vi "error_ checker.vi"() -> ()   [LabVIEW 2017]
uses:
  <vilib>/FPGAPlugInAG/myRIO-1900/niLvFpga_Open_myRIO-1900.vi
  <vilib>/rvi/interface/common/dynamic/niFpgaDynamicAddResources.vi
  <vilib>/rvi/interface/common/niFpgaWaitOnOcc.vi
  <vilib>/Utility/error.llb/Error Cluster From Error Code.vi
  <vilib>/rvi/errors/niLvFpgaAdjustHostInterfaceError.vi
  <vilib>/express/express shared/transition.llb/Dynamic To Waveform Array.vi
  <vilib>/express/express signal manip/GetorSetDDTAttributes/Set DDT Attributes/SetT0.vi
  <vilib>/express/express shared/transition.llb/Waveform Array To Dynamic.vi
  <vilib>/FPGAPlugInAG/Dynamic/niLvFpga_Close_Dynamic.vi
  <vilib>/rvi/interface/nirviOpenFPGA/nirviOpenFPGA.xnode
  FPGA Bitfiles/testznakowarki_FPGATarget_readtescior_VLrWmtzxVOU.lvbitx
  read_and_write.vi
  <vilib>/rvi/interface/nirviMethod/nirviMethod.xnode
  <vilib>/rvi/interface/nirviReadWriteControl/nirviReadWriteControl.xnode
  <vilib>/express/express signal manip/GetorSetDDTAttributes/Set DDT Attributes/Set DDT Properties.xnode
  <vilib>/rvi/interface/nirviCloseFPGA/nirviCloseFPGA.xnode
  <vilib>/rvi/errors/niLvFpgaMergeErrorWithErrorCode.vi
  <vilib>/FPGAPlugInAG/Dynamic/niLvFpga_ConfigureFifo_Dynamic.vi
  NiFpgaLv.dll
  <vilib>/rvi/interface/Simulation/niFpgaSimulationCallBeginRW.vi
  <vilib>/FPGAPlugInAG/Dynamic/niLvFpga_ReadFifo_Dynamic.vi
panel:
  in  "stop":bool
  out "?":string="this parameter determines how fast function reads data, higher value means slower reading and lower accuracy (use hundreds or thousands)"
  in  "ticks reading":u32=500
  out "Warning":string="cannot exceed 1023 and must be lower than number of pts after trigger stops (better not go under 150)"
  in  "number of elements":u32=150
  out "cycles to complete":i32
  out "gen size checker":i32
  in  "?":enum32{"now", "data", "settings"}(tab)=enum."settings"
  out "gathered error x graph":cluster{"time":i32[], "data y":i16[]}[](graph)=[{"time"=[0, 1, 2, 3, 4, 5, 6, 7, 8, 9, 10, 11, 12, 13, 14, 15, 16, 17, 18, 19, 20, 21, 22, 23, 24, 25, 26, 27, 28, 29, 30, 31, 32, 33, 34, 35, 36, 37, 38, 39, 40, 41, 42, 43, 44, 45, 46, 47, 48, 49, 50, 51, 52, 53, 54, 55, 56, 57, 58, 59, 60, 61, 62, 63, 64, 65, 66, 67, 68, 69, 70, 71, 72, 73, 74, 75, 76, 77, 78, 79, 80, 81, 82, 83, 84, 85, 86, 87, 88, 89, 90, 91, 92, 93, 94, 95, 96, 97, 98, 99, 100, 101, 102, 103, 104, 105, 106, 107, 108, 109, 110, 111, 112, 113, 114, 115, 116, 117, 118, 119, 120, 121, 122, 123, 124, 125, 126, 127, 128, 129, 130, 131, 132, 133, 134, 135, 136, 137, 138, 139, 140, 141, 142, 143, 144, 145, 146, 147, 148, 149, 150, 151, 152, 153, 154, 155, 156, 157, 158, 159, 160, 161, 162, 163, 164, 165, 166, 167, 168, 169, 170, 171, 172, 173, 174, 175, 176, 177, 178, 179, 180, 181, 182, 183, 184, 185, 186, 187, 188, 189, 190, 191, 192, 193, 194, 195, 196, 197, 198, 199, 200, 201, 202, 203, 204, 205, 206, 207, 208, 209, 210, 211, 212, 213, 214, 215, 216, 217, 218, 219, 220, 221, 222, 223, 224, 225, 226, 227, 228, 229, 230, 231, 232, 233, 234, 235, 236, 237, 238, 239, 240, 241, 242, 243, 244, 245, 246, 247, 248, 249, 250, 251, 252, 253, 254, 255, 256, 257, 258, 259, 260, 261, 262, 263, 264, 265, 266, 267, 268, 269, 270, 271, 272, 273, 274, 275, 276, 277, 278, 279, 280, 281, 282, 283, 284, 285, 286, 287, 288, 289, 290, 291, 292, 293, 294, 295, 296, 297, 298, 299], "data y"=[1986, 1970, 1920, 1858, 1861, 1860, 1808, 1774, 1734, 1748, 1695, 1675, 1665, 1650, 1668, 1624, 1652, 1624, 1636, 1627, 1647, 1655, 1677, 1675, 1696, 1728, 1732, 1725, 1767, 1796, 1796, 1846, 1885, 1873, 1909, 1930, 1975, 1952, 1993, 2008, 2014, 1986, 2017, 2037, 2018, 2020, 2017, 1998, 1997, 2030, 2037, 2018, 2013, 2029, 2019, 2007, 2043, 2014, 2019, 2007, 2050, 2067, 1998, 1985, 2043, 2057, 2007, 1991, 1987, 2004, 2037, 2047, 2025, 2039, 2020, 2050, 2026, 2017, 2027, 1996, 1995, 2047, 2055, 2019, 2007, 2022, 2029, 1994, 2029, 2067, 2028, 2005, 2024, 2042, 2033, 2047, 2027, 2005, 2016, 2041, 2018, 2017, 2008, 2015, 2025, 2052, 2056, 2042, 2049, 2011, 2005, 2043, 2052, 2027, 2021, 2058, 2051, 2038, 2045, 2022, 2015, 2048, 2058, 2047, 2061, 2024, 2039, 2035, 2055, 2055, 2022, 2037, 2039, 2014, 2036, 2053, 2025, 2054, 2042, 2058, 2034, 2044, 2063, 2042, 2023, 2043, 2027, 2039, 2067, 2063, 2047, 2011, 2045, 2057, 2037, 2051, 2049, 2016, 2038, 2064, 2038, 2041, 2053, 2027, 2045, 2040, 2064, 2037, 2020, 2047, 2047, 2032, 2068, 2049, 2023, 2035, 2043, 2081, 2038, 2041, 2045, 2010, 2028, 2059, 2045, 2050, 2067, 2035, 2035, 2059, 2051, 2040, 2025, 2051, 2052, 2031, 2063, 2062, 2027, 2051, 2054, 2022, 2036, 2040, 2057, 2037, 2048, 2064, 2038, 2033, 2058, 2045, 2037, 2051, 2027, 2053, 2025, 2031, 2033, 2023, 2049, 2053, 2038, 2054, 2050, 2025, 2041, 2067, 2039, 2016, 2030, 2056, 2045, 2052, 2067, 2029, 2027, 2045, 2023, 2031, 2065, 2065, 2053, 2041, 2057, 2037, 2017, 2027, 2027, 2028, 2064, 2078, 2042, 2045, 2036, 2069, 2043, 2032, 2038, 2018, 2047, 2072, 2041, 2045, 2053, 2026, 2030, 2016, 2034, 2023, 2025, 2065, 2047, 2029, 2041, 2029, 2032, 2067, 2054, 2031, 2051, 2067, 2051, 2016, 2036, 2063, 2047, 2060, 2064, 2026, 2024, 2045, 2026, 2028, 2012, 2034, 2026, 2031, 2055, 2041]}, {"time"=[0, 1, 2, 3, 4, 5, 6, 7, 8, 9, 10, 11, 12, 13, 14, 15, 16, 17, 18, 19, 20, 21, 22, 23, 24, 25, 26, 27, 28, 29, 30, 31, 32, 33, 34, 35, 36, 37, 38, 39, 40, 41, 42, 43, 44, 45, 46, 47, 48, 49, 50, 51, 52, 53, 54, 55, 56, 57, 58, 59, 60, 61, 62, 63, 64, 65, 66, 67, 68, 69, 70, 71, 72, 73, 74, 75, 76, 77, 78, 79, 80, 81, 82, 83, 84, 85, 86, 87, 88, 89, 90, 91, 92, 93, 94, 95, 96, 97, 98, 99, 100, 101, 102, 103, 104, 105, 106, 107, 108, 109, 110, 111, 112, 113, 114, 115, 116, 117, 118, 119, 120, 121, 122, 123, 124, 125, 126, 127, 128, 129, 130, 131, 132, 133, 134, 135, 136, 137, 138, 139, 140, 141, 142, 143, 144, 145, 146, 147, 148, 149, 150, 151, 152, 153, 154, 155, 156, 157, 158, 159, 160, 161, 162, 163, 164, 165, 166, 167, 168, 169, 170, 171, 172, 173, 174, 175, 176, 177, 178, 179, 180, 181, 182, 183, 184, 185, 186, 187, 188, 189, 190, 191, 192, 193, 194, 195, 196, 197, 198, 199, 200, 201, 202, 203, 204, 205, 206, 207, 208, 209, 210, 211, 212, 213, 214, 215, 216, 217, 218, 219, 220, 221, 222, 223, 224, 225, 226, 227, 228, 229, 230, 231, 232, 233, 234, 235, 236, 237, 238, 239, 240, 241, 242, 243, 244, 245, 246, 247, 248, 249, 250, 251, 252, 253, 254, 255, 256, 257, 258, 259, 260, 261, 262, 263, 264, 265, 266, 267, 268, 269, 270, 271, 272, 273, 274, 275, 276, 277, 278, 279, 280, 281, 282, 283, 284, 285, 286, 287, 288, 289, 290, 291, 292, 293, 294, 295, 296, 297, 298, 299], "data y"=[2382, 2659, 2664, 2672, 2666, 2654, 2660, 2664, 2667, 2655, 2663, 2668, 2662, 2667, 2660, 2658, 2661, 2670, 2657, 2659, 2671, 2214, 1624, 1315, 1097, 961, 861, 782, 703, 622, 628, 628, 621, 632, 635, 636, 668, 754, 892, 1012, 1172, 1362, 1513, 1661, 1801, 1899, 1955, 2029, 2076, 2101, 2109, 2111, 2110, 2082, 2059, 2050, 2019, 2037, 2053, 2067, 2089, 2092, 2091, 2116, 2097, 2066, 2077, 2087, 2092, 2091, 2075, 2066, 2058, 2046, 2042, 2030, 2048, 2065, 2051, 2053, 2073, 2052, 2041, 2052, 2058, 2057, 2062, 2070, 2067, 2039, 2044, 2048, 2041, 2035, 2026, 2037, 2059, 2060, 2064, 2055, 2051, 2045, 2046, 2067, 2066, 2040, 2041, 2052, 2045, 2056, 2059, 2044, 2042, 2049, 2042, 2045, 2048, 2064, 2060, 2052, 2064, 2055, 2049, 2055, 2038, 2049, 2038, 2059, 2059, 2059, 2053, 2052, 2046, 2056, 2051, 2029, 2043, 2048, 2054, 2041, 2058, 2056, 2039, 2045, 2065, 2054, 2055, 2056, 2040, 2049, 2055, 2052, 2042, 2044, 2058, 2064, 2055, 2068, 2065, 2050, 2052, 2058, 2039, 2040, 2037, 2050, 2054, 2060, 2067, 2043, 2053, 2057, 2047, 2037, 2050, 2054, 2047, 2035, 2047, 2063, 2052, 2061, 2064, 2047, 2055, 2066, 2056, 2062, 2068, 2061, 2042, 2035, 2047, 2037, 2034, 2043, 2046, 2039, 2053, 2058, 2051, 2070, 2063, 2056, 2042, 2055, 2069, 2039, 2044, 2052, 2049, 2048, 2061, 2059, 2057, 2043, 2058, 2052, 2041, 2054, 2044, 2038, 2048, 2045, 2043, 2072, 2072, 2057, 2058, 2056, 2063, 2049, 2054, 2056, 2047, 2046, 2059, 2041, 2042, 2055, 2052, 2045, 2045, 2059, 2050, 2057, 2068, 2054, 2051, 2057, 2041, 2031, 2051, 2048, 2056, 2040, 2050, 2056, 2045, 2062, 2059, 2035, 2032, 2053, 2042, 2056, 2063, 2063, 2048, 2052, 2065, 2057, 2044, 2053, 2053, 2043, 2050, 2058, 2035, 2058, 2049, 2058, 2047, 2056, 2061, 2045, 2052, 2054, 2042, 2051, 2051, 2056, 2062, 2047, 2066, 2048, 2050, 2062, 2056, 2049]}]
  out "gathered error y graph":cluster{"time":i32[], "data y":i16[]}[](graph)=[{"time"=[0, 1, 2, 3, 4, 5, 6, 7, 8, 9, 10, 11, 12, 13, 14, 15, 16, 17, 18, 19, 20, 21, 22, 23, 24, 25, 26, 27, 28, 29, 30, 31, 32, 33, 34, 35, 36, 37, 38, 39, 40, 41, 42, 43, 44, 45, 46, 47, 48, 49, 50, 51, 52, 53, 54, 55, 56, 57, 58, 59, 60, 61, 62, 63, 64, 65, 66, 67, 68, 69, 70, 71, 72, 73, 74, 75, 76, 77, 78, 79, 80, 81, 82, 83, 84, 85, 86, 87, 88, 89, 90, 91, 92, 93, 94, 95, 96, 97, 98, 99, 100, 101, 102, 103, 104, 105, 106, 107, 108, 109, 110, 111, 112, 113, 114, 115, 116, 117, 118, 119, 120, 121, 122, 123, 124, 125, 126, 127, 128, 129, 130, 131, 132, 133, 134, 135, 136, 137, 138, 139, 140, 141, 142, 143, 144, 145, 146, 147, 148, 149, 150, 151, 152, 153, 154, 155, 156, 157, 158, 159, 160, 161, 162, 163, 164, 165, 166, 167, 168, 169, 170, 171, 172, 173, 174, 175, 176, 177, 178, 179, 180, 181, 182, 183, 184, 185, 186, 187, 188, 189, 190, 191, 192, 193, 194, 195, 196, 197, 198, 199, 200, 201, 202, 203, 204, 205, 206, 207, 208, 209, 210, 211, 212, 213, 214, 215, 216, 217, 218, 219, 220, 221, 222, 223, 224, 225, 226, 227, 228, 229, 230, 231, 232, 233, 234, 235, 236, 237, 238, 239, 240, 241, 242, 243, 244, 245, 246, 247, 248, 249, 250, 251, 252, 253, 254, 255, 256, 257, 258, 259, 260, 261, 262, 263, 264, 265, 266, 267, 268, 269, 270, 271, 272, 273, 274, 275, 276, 277, 278, 279, 280, 281, 282, 283, 284, 285, 286, 287, 288, 289, 290, 291, 292, 293, 294, 295, 296, 297, 298, 299], "data y"=[2052, 2061, 2063, 2041, 2035, 2058, 2066, 2066, 2068, 2062, 2054, 2045, 2073, 2074, 2031, 2080, 2051, 2055, 2053, 2054, 2043, 2050, 2071, 2049, 2039, 2046, 2056, 2052, 2059, 2073, 2060, 2061, 2059, 2053, 2058, 2041, 2063, 2064, 2041, 2074, 2068, 2060, 2061, 2064, 2053, 2064, 2069, 2050, 2057, 2054, 2058, 2068, 2050, 2066, 2058, 2050, 2048, 2081, 2035, 2068, 2067, 2055, 2041, 2070, 2087, 2039, 2024, 2054, 2084, 2074, 2072, 2075, 2054, 2050, 2042, 2059, 2070, 2058, 2070, 2066, 2030, 2041, 2074, 2068, 2051, 2046, 2038, 2042, 2033, 2063, 2075, 2051, 2043, 2045, 2055, 2072, 2070, 2055, 2048, 2075, 2054, 2057, 2058, 2055, 2044, 2046, 2064, 2059, 2068, 2056, 2038, 2052, 2062, 2062, 2038, 2053, 2076, 2054, 2060, 2063, 2037, 2046, 2061, 2046, 2058, 2035, 2053, 2046, 2052, 2063, 2052, 2047, 2059, 2040, 2038, 2060, 2050, 2050, 2053, 2059, 2052, 2039, 2063, 2065, 2052, 2055, 2054, 2039, 2056, 2066, 2056, 2029, 2034, 2060, 2058, 2056, 2072, 2053, 2039, 2055, 2052, 2045, 2060, 2057, 2065, 2049, 2063, 2074, 2046, 2047, 2055, 2032, 2047, 2072, 2051, 2051, 2066, 2072, 2070, 2051, 2059, 2046, 2032, 2047, 2057, 2052, 2073, 2073, 2049, 2057, 2053, 2063, 2048, 2046, 2064, 2046, 2057, 2075, 2056, 2049, 2067, 2045, 2041, 2046, 2059, 2061, 2046, 2060, 2055, 2037, 2051, 2062, 2055, 2063, 2060, 2080, 2051, 2046, 2047, 2029, 2038, 2060, 2054, 2060, 2074, 2052, 2047, 2053, 2057, 2048, 2032, 2054, 2054, 2047, 2064, 2059, 2037, 2043, 2051, 2044, 2065, 2045, 2059, 2050, 2065, 2071, 2047, 2042, 2047, 2033, 2042, 2064, 2058, 2053, 2031, 2065, 2064, 2049, 2059, 2047, 2044, 2053, 2059, 2053, 2069, 2059, 2033, 2041, 2045, 2053, 2035, 2046, 2064, 2045, 2051, 2058, 2041, 2052, 2068, 2054, 2055, 2060, 2071, 2055, 2038, 2060, 2052, 2047, 2069, 2058, 2042, 2056, 2049, 2066, 2040, 2050, 2056, 2034, 2055, 2059]}, {"time"=[0, 1, 2, 3, 4, 5, 6, 7, 8, 9, 10, 11, 12, 13, 14, 15, 16, 17, 18, 19, 20, 21, 22, 23, 24, 25, 26, 27, 28, 29, 30, 31, 32, 33, 34, 35, 36, 37, 38, 39, 40, 41, 42, 43, 44, 45, 46, 47, 48, 49, 50, 51, 52, 53, 54, 55, 56, 57, 58, 59, 60, 61, 62, 63, 64, 65, 66, 67, 68, 69, 70, 71, 72, 73, 74, 75, 76, 77, 78, 79, 80, 81, 82, 83, 84, 85, 86, 87, 88, 89, 90, 91, 92, 93, 94, 95, 96, 97, 98, 99, 100, 101, 102, 103, 104, 105, 106, 107, 108, 109, 110, 111, 112, 113, 114, 115, 116, 117, 118, 119, 120, 121, 122, 123, 124, 125, 126, 127, 128, 129, 130, 131, 132, 133, 134, 135, 136, 137, 138, 139, 140, 141, 142, 143, 144, 145, 146, 147, 148, 149, 150, 151, 152, 153, 154, 155, 156, 157, 158, 159, 160, 161, 162, 163, 164, 165, 166, 167, 168, 169, 170, 171, 172, 173, 174, 175, 176, 177, 178, 179, 180, 181, 182, 183, 184, 185, 186, 187, 188, 189, 190, 191, 192, 193, 194, 195, 196, 197, 198, 199, 200, 201, 202, 203, 204, 205, 206, 207, 208, 209, 210, 211, 212, 213, 214, 215, 216, 217, 218, 219, 220, 221, 222, 223, 224, 225, 226, 227, 228, 229, 230, 231, 232, 233, 234, 235, 236, 237, 238, 239, 240, 241, 242, 243, 244, 245, 246, 247, 248, 249, 250, 251, 252, 253, 254, 255, 256, 257, 258, 259, 260, 261, 262, 263, 264, 265, 266, 267, 268, 269, 270, 271, 272, 273, 274, 275, 276, 277, 278, 279, 280, 281, 282, 283, 284, 285, 286, 287, 288, 289, 290, 291, 292, 293, 294, 295, 296, 297, 298, 299], "data y"=[2038, 2035, 2029, 2040, 2046, 2033, 2032, 2044, 2045, 2051, 2047, 2071, 2062, 2041, 2051, 2057, 2045, 2056, 2044, 2031, 2045, 2055, 2077, 2043, 2027, 2024, 2008, 2031, 2040, 2035, 2041, 2047, 2038, 2036, 2058, 2071, 2043, 2042, 2051, 2057, 2038, 2058, 2064, 2032, 2042, 2053, 2038, 2035, 2028, 2043, 2031, 2041, 2046, 2044, 2028, 2042, 2034, 2027, 2025, 2040, 2014, 2026, 2051, 2058, 2041, 2044, 2072, 2066, 2044, 2037, 2040, 2038, 2050, 2052, 2053, 2048, 2038, 2045, 2049, 2031, 2056, 2055, 2035, 2034, 2051, 2053, 2052, 2037, 2060, 2043, 2027, 2029, 2040, 2037, 2028, 2041, 2035, 2024, 2049, 2039, 2034, 2036, 2030, 2050, 2050, 2042, 2036, 2041, 2036, 2038, 2041, 2030, 2043, 2044, 2053, 2056, 2047, 2055, 2049, 2029, 2034, 2048, 2041, 2044, 2050, 2044, 2036, 2047, 2050, 2022, 2023, 2032, 2040, 2034, 2051, 2043, 2039, 2044, 2052, 2049, 2040, 2048, 2033, 2021, 2034, 2032, 2026, 2049, 2051, 2034, 2049, 2054, 2055, 2045, 2049, 2058, 2048, 2048, 2057, 2047, 2044, 2046, 2037, 2032, 2044, 2043, 2042, 2032, 2034, 2048, 2045, 2053, 2054, 2031, 2015, 2032, 2032, 2030, 2030, 2033, 2039, 2045, 2062, 2048, 2044, 2052, 2047, 2027, 2037, 2043, 2049, 2047, 2051, 2046, 2033, 2036, 2036, 2037, 2042, 2055, 2035, 2032, 2038, 2037, 2035, 2038, 2060, 2053, 2043, 2046, 2047, 2045, 2048, 2042, 2041, 2026, 2028, 2049, 2045, 2045, 2052, 2041, 2038, 2036, 2027, 2029, 2047, 2045, 2034, 2051, 2081, 2094, 2083, 2101, 2093, 2078, 2070, 2061, 2036, 2027, 2027, 2036, 2012, 2002, 2022, 2018, 2024, 2027, 2021, 2021, 2036, 2025, 2035, 2036, 2026, 2039, 2024, 2029, 2031, 2039, 2062, 2048, 2038, 2039, 2042, 2041, 2055, 2036, 2039, 2029, 2045, 2055, 2034, 2033, 2041, 2037, 2056, 2052, 2037, 2027, 2027, 2038, 2036, 2038, 2050, 2061, 2054, 2046, 2028, 2029, 2036, 2040, 2034, 2027, 2028, 2037, 2025, 2050, 2048, 2041]}]
  out "error x graph current elements":cluster{"time":i32[], "data y":i16[]}[](graph)=[{"time"=[0, 1, 2, 3, 4, 5, 6, 7, 8, 9, 10, 11, 12, 13, 14, 15, 16, 17, 18, 19, 20, 21, 22, 23, 24, 25, 26, 27, 28, 29, 30, 31, 32, 33, 34, 35, 36, 37, 38, 39, 40, 41, 42, 43, 44, 45, 46, 47, 48, 49, 50, 51, 52, 53, 54, 55, 56, 57, 58, 59, 60, 61, 62, 63, 64, 65, 66, 67, 68, 69, 70, 71, 72, 73, 74, 75, 76, 77, 78, 79, 80, 81, 82, 83, 84, 85, 86, 87, 88, 89, 90, 91, 92, 93, 94, 95, 96, 97, 98, 99, 100, 101, 102, 103, 104, 105, 106, 107, 108, 109, 110, 111, 112, 113, 114, 115, 116, 117, 118, 119, 120, 121, 122, 123, 124, 125, 126, 127, 128, 129, 130, 131, 132, 133, 134, 135, 136, 137, 138, 139, 140, 141, 142, 143, 144, 145, 146, 147, 148, 149], "data y"=[2071, 2039, 2036, 2051, 2051, 2040, 2029, 2062, 2055, 2035, 2053, 2044, 2025, 2060, 2073, 2030, 2042, 2039, 2050, 2027, 2018, 2046, 2065, 2037, 2057, 2053, 2030, 2049, 2072, 2034, 2032, 2069, 2083, 2035, 2030, 2040, 2024, 2055, 2070, 2033, 2041, 2049, 2031, 2029, 2032, 2062, 2045, 2038, 2054, 2026, 2016, 2048, 2049, 2056, 2084, 2060, 2040, 2028, 2066, 2074, 2043, 2052, 2055, 2015, 2037, 2057, 2029, 2048, 2069, 2071, 2045, 2044, 2061, 2031, 2028, 2050, 2031, 2019, 2047, 2042, 2042, 2005, 2029, 2053, 2044, 2072, 2074, 2039, 2044, 2049, 2016, 2032, 2063, 2045, 2044, 2043, 2073, 2063, 2043, 2058, 2045, 2025, 2047, 2057, 2042, 2063, 2066, 2051, 2019, 2033, 2062, 2055, 2062, 2069, 2033, 2017, 2035, 2015, 2027, 2069, 2055, 2051, 2026, 2055, 2066, 2026, 2042, 2049, 2025, 2052, 2074, 2037, 2052, 2032, 2052, 2038, 2035, 2071, 2063, 2047, 2063, 2041, 2011, 2026, 2048, 2036, 2023, 2027, 2061, 2046]}, {"time"=[0, 1, 2, 3, 4, 5, 6, 7, 8, 9, 10, 11, 12, 13, 14, 15, 16, 17, 18, 19, 20, 21, 22, 23, 24, 25, 26, 27, 28, 29, 30, 31, 32, 33, 34, 35, 36, 37, 38, 39, 40, 41, 42, 43, 44, 45, 46, 47, 48, 49, 50, 51, 52, 53, 54, 55, 56, 57, 58, 59, 60, 61, 62, 63, 64, 65, 66, 67, 68, 69, 70, 71, 72, 73, 74, 75, 76, 77, 78, 79, 80, 81, 82, 83, 84, 85, 86, 87, 88, 89, 90, 91, 92, 93, 94, 95, 96, 97, 98, 99, 100, 101, 102, 103, 104, 105, 106, 107, 108, 109, 110, 111, 112, 113, 114, 115, 116, 117, 118, 119, 120, 121, 122, 123, 124, 125, 126, 127, 128, 129, 130, 131, 132, 133, 134, 135, 136, 137, 138, 139, 140, 141, 142, 143, 144, 145, 146, 147, 148, 149], "data y"=[2031, 2054, 2044, 2020, 2028, 2026, 2038, 2032, 2038, 2052, 2051, 2045, 2052, 2046, 2035, 2047, 2043, 2036, 2028, 2038, 2051, 2042, 2033, 2029, 2035, 2043, 2060, 2055, 2033, 2037, 2044, 2041, 2039, 2042, 2048, 2039, 2050, 2042, 2030, 2039, 2042, 2034, 2037, 2048, 2059, 2039, 2035, 2035, 2032, 2041, 2051, 2038, 2036, 2039, 2045, 2042, 2042, 2049, 2028, 2031, 2036, 2041, 2048, 2056, 2048, 2025, 2034, 2037, 2026, 2042, 2045, 2058, 2040, 2028, 2043, 2033, 2039, 2064, 2056, 2046, 2052, 2042, 2039, 2027, 2041, 2048, 2036, 2049, 2056, 2047, 2047, 2043, 2028, 2039, 2046, 2058, 2039, 2033, 2035, 2035, 2033, 2043, 2035, 2040, 2053, 2050, 2049, 2045, 2044, 2051, 2030, 2038, 2051, 2038, 2047, 2050, 2040, 2047, 2055, 2033, 2055, 2049, 2049, 2041, 2033, 2045, 2042, 2033, 2050, 2058, 2042, 2049, 2050, 2049, 2036, 2041, 2047, 2039, 2041, 2053, 2036, 2043, 2053, 2048, 2040, 2050, 2049, 2055, 2042, 2037]}]
  out "error y graph current elements":cluster{"time":i32[], "data y":i16[]}[](graph)=[{"time"=[0, 1, 2, 3, 4, 5, 6, 7, 8, 9, 10, 11, 12, 13, 14, 15, 16, 17, 18, 19, 20, 21, 22, 23, 24, 25, 26, 27, 28, 29, 30, 31, 32, 33, 34, 35, 36, 37, 38, 39, 40, 41, 42, 43, 44, 45, 46, 47, 48, 49, 50, 51, 52, 53, 54, 55, 56, 57, 58, 59, 60, 61, 62, 63, 64, 65, 66, 67, 68, 69, 70, 71, 72, 73, 74, 75, 76, 77, 78, 79, 80, 81, 82, 83, 84, 85, 86, 87, 88, 89, 90, 91, 92, 93, 94, 95, 96, 97, 98, 99, 100, 101, 102, 103, 104, 105, 106, 107, 108, 109, 110, 111, 112, 113, 114, 115, 116, 117, 118, 119, 120, 121, 122, 123, 124, 125, 126, 127, 128, 129, 130, 131, 132, 133, 134, 135, 136, 137, 138, 139, 140, 141, 142, 143, 144, 145, 146, 147, 148, 149], "data y"=[2068, 2051, 2035, 2052, 2049, 2060, 2029, 2046, 2069, 2056, 2055, 2055, 2034, 2045, 2070, 2055, 2046, 2047, 2067, 2061, 2039, 2034, 2051, 2048, 2059, 2067, 2047, 2037, 2058, 2053, 2044, 2042, 2066, 2060, 2043, 2052, 2037, 2041, 2051, 2043, 2030, 2050, 2044, 2054, 2036, 2047, 2055, 2042, 2056, 2057, 2036, 2045, 2054, 2043, 2057, 2072, 2051, 2030, 2044, 2068, 2059, 2056, 2065, 2042, 2029, 2050, 2042, 2040, 2065, 2054, 2061, 2038, 2053, 2055, 2032, 2055, 2061, 2039, 2046, 2053, 2030, 2036, 2029, 2049, 2043, 2052, 2074, 2061, 2048, 2058, 2043, 2028, 2047, 2053, 2057, 2039, 2049, 2063, 2043, 2056, 2063, 2047, 2046, 2059, 2049, 2050, 2059, 2060, 2049, 2034, 2049, 2053, 2047, 2070, 2063, 2039, 2041, 2042, 2025, 2049, 2052, 2060, 2032, 2037, 2059, 2052, 2039, 2062, 2048, 2041, 2066, 2056, 2037, 2038, 2052, 2060, 2035, 2053, 2072, 2053, 2060, 2068, 2041, 2035, 2049, 2037, 2055, 2034, 2042, 2055]}, {"time"=[0, 1, 2, 3, 4, 5, 6, 7, 8, 9, 10, 11, 12, 13, 14, 15, 16, 17, 18, 19, 20, 21, 22, 23, 24, 25, 26, 27, 28, 29, 30, 31, 32, 33, 34, 35, 36, 37, 38, 39, 40, 41, 42, 43, 44, 45, 46, 47, 48, 49, 50, 51, 52, 53, 54, 55, 56, 57, 58, 59, 60, 61, 62, 63, 64, 65, 66, 67, 68, 69, 70, 71, 72, 73, 74, 75, 76, 77, 78, 79, 80, 81, 82, 83, 84, 85, 86, 87, 88, 89, 90, 91, 92, 93, 94, 95, 96, 97, 98, 99, 100, 101, 102, 103, 104, 105, 106, 107, 108, 109, 110, 111, 112, 113, 114, 115, 116, 117, 118, 119, 120, 121, 122, 123, 124, 125, 126, 127, 128, 129, 130, 131, 132, 133, 134, 135, 136, 137, 138, 139, 140, 141, 142, 143, 144, 145, 146, 147, 148, 149], "data y"=[2036, 2036, 2036, 2027, 2041, 2049, 2053, 2045, 2033, 2036, 2043, 2038, 2041, 2048, 2028, 2040, 2061, 2051, 2042, 2027, 2042, 2055, 2032, 2026, 2042, 2037, 2044, 2064, 2046, 2027, 2053, 2049, 2046, 2037, 2047, 2043, 2044, 2047, 2049, 2045, 2040, 2031, 2039, 2038, 2048, 2055, 2031, 2025, 2025, 2033, 2046, 2051, 2054, 2062, 2044, 2036, 2035, 2046, 2045, 2033, 2038, 2042, 2047, 2053, 2058, 2046, 2052, 2052, 2037, 2051, 2037, 2042, 2043, 2029, 2034, 2039, 2029, 2043, 2049, 2048, 2050, 2035, 2049, 2049, 2043, 2046, 2036, 2040, 2042, 2032, 2033, 2056, 2049, 2019, 2046, 2056, 2058, 2047, 2045, 2045, 2034, 2038, 2048, 2050, 2056, 2054, 2032, 2033, 2038, 2040, 2045, 2035, 2051, 2045, 2031, 2038, 2045, 2042, 2048, 2050, 2057, 2042, 2040, 2054, 2042, 2031, 2038, 2040, 2030, 2051, 2047, 2044, 2060, 2046, 2035, 2026, 2044, 2039, 2042, 2048, 2059, 2053, 2042, 2047, 2051, 2047, 2029, 2049, 2046, 2037]}]
  out "template graph x":cluster{"time":i32[], "data y":i16[]}[](graph)=[{"time"=[0, 1, 2, 3, 4, 5, 6, 7, 8, 9, 10, 11, 12, 13, 14, 15, 16, 17, 18, 19, 20, 21, 22, 23, 24, 25, 26, 27, 28, 29, 30, 31, 32, 33, 34, 35, 36, 37, 38, 39, 40, 41, 42, 43, 44, 45, 46, 47, 48, 49, 50, 51, 52, 53, 54, 55, 56, 57, 58, 59, 60, 61, 62, 63, 64, 65, 66, 67, 68, 69, 70, 71, 72, 73, 74, 75, 76, 77, 78, 79, 80, 81, 82, 83, 84, 85, 86, 87, 88, 89, 90, 91, 92, 93, 94, 95, 96, 97, 98, 99, 100, 101, 102, 103, 104, 105, 106, 107, 108, 109, 110, 111, 112, 113, 114, 115, 116, 117, 118, 119, 120, 121, 122, 123, 124, 125, 126, 127, 128, 129, 130, 131, 132, 133, 134, 135, 136, 137, 138, 139, 140, 141, 142, 143, 144, 145, 146, 147, 148, 149, 150, 151, 152, 153, 154, 155, 156, 157, 158, 159, 160, 161, 162, 163, 164, 165, 166, 167, 168, 169, 170, 171, 172, 173, 174, 175, 176, 177, 178, 179, 180, 181, 182, 183, 184, 185, 186, 187, 188, 189, 190, 191, 192, 193, 194, 195, 196, 197, 198, 199, 200, 201, 202, 203, 204, 205, 206, 207, 208, 209, 210, 211, 212, 213, 214, 215, 216, 217, 218, 219, 220, 221, 222, 223, 224, 225, 226, 227, 228, 229, 230, 231, 232, 233, 234, 235, 236, 237, 238, 239, 240, 241, 242, 243, 244, 245, 246, 247, 248, 249, 250, 251, 252, 253, 254, 255, 256, 257, 258, 259, 260, 261, 262, 263, 264, 265, 266, 267, 268, 269, 270, 271, 272, 273, 274, 275, 276, 277, 278, 279, 280, 281, 282, 283, 284, 285, 286, 287, 288, 289, 290, 291, 292, 293, 294, 295, 296, 297, 298, 299], "data y"=[1987, 1971, 1955, 1885, 1866, 1853, 1810, 1748, 1734, 1732, 1693, 1670, 1650, 1620, 1668, 1631, 1633, 1604, 1653, 1636, 1640, 1666, 1683, 1678, 1678, 1708, 1728, 1718, 1749, 1797, 1795, 1816, 1846, 1904, 1919, 1903, 1949, 1977, 1957, 2028, 2013, 1998, 2012, 2026, 2009, 2022, 2026, 2052, 2031, 2007, 2043, 2018, 2015, 2033, 2040, 1992, 2027, 2023, 2033, 2030, 1985, 2043, 2038, 1979, 2014, 2055, 2048, 2007, 1978, 1979, 2011, 1998, 2018, 2016, 2008, 2028, 2038, 2005, 2018, 2031, 2005, 2038, 2052, 2009, 2023, 2027, 2046, 2020, 2020, 2044, 2019, 2027, 2049, 2016, 2006, 2046, 2025, 2014, 2006, 2032, 2035, 2051, 2066, 2024, 2004, 2035, 2037, 2024, 2053, 2028, 2035, 2032, 2053, 2061, 2024, 2034, 2050, 2011, 2030, 2053, 2036, 2023, 2037, 2053, 2038, 2015, 2038, 2049, 2038, 2057, 2054, 2015, 2040, 2055, 2035, 2017, 2023, 2059, 2050, 2052, 2074, 2039, 2027, 2049, 2031, 2026, 2058, 2069, 2056, 2031, 2058, 2069, 2027, 2018, 2049, 2031, 2034, 2067, 2053, 2042, 2059, 2039, 2051, 2027, 2047, 2065, 2031, 2036, 2064, 2048, 2042, 2060, 2048, 2026, 2027, 2058, 2069, 2034, 2041, 2059, 2032, 2054, 2071, 2037, 2035, 2032, 2034, 2065, 2038, 2032, 2036, 2027, 2025, 2055, 2029, 2029, 2058, 2039, 2033, 2063, 2047, 2035, 2014, 2039, 2033, 2022, 2058, 2042, 2024, 2053, 2049, 2027, 2053, 2041, 2041, 2021, 2048, 2055, 2028, 2045, 2047, 2020, 2031, 2042, 2020, 2027, 2034, 2057, 2036, 2044, 2065, 2026, 2014, 2035, 2030, 2024, 2058, 2040, 2042, 2025, 2048, 2055, 2032, 2042, 2053, 2024, 2042, 2072, 2053, 2054, 2054, 2066, 2045, 2045, 2063, 2039, 2026, 2044, 2030, 2020, 2052, 2039, 2019, 2053, 2034, 2046, 2022, 2057, 2077, 2044, 2045, 2048, 2019, 2031, 2049, 2026, 2027, 2032, 2049, 2029, 2009, 2046, 2052, 2051, 2080, 2061, 2033, 2040, 2029, 2012, 2032, 2044, 2065, 2034, 2037, 2056, 2031, 2042, 2072, 2046]}, {"time"=[0, 1, 2, 3, 4, 5, 6, 7, 8, 9, 10, 11, 12, 13, 14, 15, 16, 17, 18, 19, 20, 21, 22, 23, 24, 25, 26, 27, 28, 29, 30, 31, 32, 33, 34, 35, 36, 37, 38, 39, 40, 41, 42, 43, 44, 45, 46, 47, 48, 49, 50, 51, 52, 53, 54, 55, 56, 57, 58, 59, 60, 61, 62, 63, 64, 65, 66, 67, 68, 69, 70, 71, 72, 73, 74, 75, 76, 77, 78, 79, 80, 81, 82, 83, 84, 85, 86, 87, 88, 89, 90, 91, 92, 93, 94, 95, 96, 97, 98, 99, 100, 101, 102, 103, 104, 105, 106, 107, 108, 109, 110, 111, 112, 113, 114, 115, 116, 117, 118, 119, 120, 121, 122, 123, 124, 125, 126, 127, 128, 129, 130, 131, 132, 133, 134, 135, 136, 137, 138, 139, 140, 141, 142, 143, 144, 145, 146, 147, 148, 149, 150, 151, 152, 153, 154, 155, 156, 157, 158, 159, 160, 161, 162, 163, 164, 165, 166, 167, 168, 169, 170, 171, 172, 173, 174, 175, 176, 177, 178, 179, 180, 181, 182, 183, 184, 185, 186, 187, 188, 189, 190, 191, 192, 193, 194, 195, 196, 197, 198, 199, 200, 201, 202, 203, 204, 205, 206, 207, 208, 209, 210, 211, 212, 213, 214, 215, 216, 217, 218, 219, 220, 221, 222, 223, 224, 225, 226, 227, 228, 229, 230, 231, 232, 233, 234, 235, 236, 237, 238, 239, 240, 241, 242, 243, 244, 245, 246, 247, 248, 249, 250, 251, 252, 253, 254, 255, 256, 257, 258, 259, 260, 261, 262, 263, 264, 265, 266, 267, 268, 269, 270, 271, 272, 273, 274, 275, 276, 277, 278, 279, 280, 281, 282, 283, 284, 285, 286, 287, 288, 289, 290, 291, 292, 293, 294, 295, 296, 297, 298, 299], "data y"=[2274, 2661, 2656, 2670, 2664, 2659, 2660, 2663, 2671, 2660, 2661, 2665, 2662, 2671, 2670, 2652, 2672, 2662, 2664, 2661, 2536, 2114, 1733, 1378, 1144, 991, 891, 826, 740, 646, 631, 634, 626, 621, 629, 644, 660, 754, 876, 1004, 1154, 1319, 1494, 1608, 1738, 1913, 1993, 2036, 2074, 2107, 2096, 2091, 2094, 2073, 2052, 2044, 2041, 2029, 2058, 2070, 2099, 2101, 2082, 2103, 2102, 2076, 2063, 2070, 2099, 2107, 2095, 2067, 2066, 2055, 2044, 2046, 2042, 2063, 2063, 2042, 2058, 2045, 2047, 2048, 2053, 2065, 2056, 2055, 2059, 2040, 2053, 2049, 2035, 2046, 2051, 2052, 2047, 2037, 2062, 2057, 2043, 2051, 2043, 2052, 2058, 2049, 2055, 2056, 2044, 2047, 2039, 2056, 2042, 2033, 2052, 2065, 2051, 2055, 2064, 2046, 2044, 2050, 2062, 2041, 2041, 2060, 2054, 2045, 2065, 2043, 2034, 2051, 2056, 2051, 2068, 2050, 2045, 2038, 2047, 2056, 2041, 2045, 2057, 2052, 2059, 2059, 2052, 2043, 2058, 2068, 2062, 2051, 2045, 2061, 2044, 2050, 2055, 2048, 2047, 2054, 2043, 2050, 2040, 2044, 2045, 2046, 2052, 2060, 2051, 2045, 2055, 2047, 2056, 2071, 2049, 2052, 2049, 2062, 2063, 2064, 2065, 2067, 2041, 2046, 2048, 2033, 2044, 2032, 2052, 2057, 2060, 2049, 2053, 2039, 2046, 2056, 2045, 2052, 2060, 2059, 2042, 2042, 2049, 2045, 2043, 2055, 2054, 2053, 2065, 2056, 2054, 2061, 2047, 2055, 2042, 2059, 2051, 2037, 2046, 2054, 2049, 2059, 2056, 2039, 2040, 2048, 2058, 2055, 2062, 2066, 2046, 2057, 2069, 2056, 2041, 2046, 2040, 2037, 2043, 2059, 2050, 2042, 2049, 2057, 2052, 2046, 2038, 2030, 2043, 2066, 2054, 2046, 2051, 2060, 2041, 2046, 2053, 2056, 2047, 2051, 2052, 2048, 2065, 2057, 2066, 2045, 2048, 2060, 2047, 2052, 2069, 2054, 2057, 2066, 2042, 2051, 2057, 2053, 2040, 2040, 2048, 2053, 2040, 2046, 2049, 2048, 2068, 2064, 2065, 2055, 2060, 2063, 2048, 2057, 2054, 2046, 2061, 2042, 2022, 2044]}]
  out "trigger count":i16=18
  out "trigger":bool
  out "template":bool=TRUE
  out "deviation error y3":bool
  out "deviation error x3":bool
  out "max/min y3":bool
  out "max/min x3":bool
  out "error y3":bool
  out "error x3":bool
  out "?":string="error now"
  out "template graph y":cluster{"time":i32[], "data y":i16[]}[](graph)=[{"time"=[0, 1, 2, 3, 4, 5, 6, 7, 8, 9, 10, 11, 12, 13, 14, 15, 16, 17, 18, 19, 20, 21, 22, 23, 24, 25, 26, 27, 28, 29, 30, 31, 32, 33, 34, 35, 36, 37, 38, 39, 40, 41, 42, 43, 44, 45, 46, 47, 48, 49, 50, 51, 52, 53, 54, 55, 56, 57, 58, 59, 60, 61, 62, 63, 64, 65, 66, 67, 68, 69, 70, 71, 72, 73, 74, 75, 76, 77, 78, 79, 80, 81, 82, 83, 84, 85, 86, 87, 88, 89, 90, 91, 92, 93, 94, 95, 96, 97, 98, 99, 100, 101, 102, 103, 104, 105, 106, 107, 108, 109, 110, 111, 112, 113, 114, 115, 116, 117, 118, 119, 120, 121, 122, 123, 124, 125, 126, 127, 128, 129, 130, 131, 132, 133, 134, 135, 136, 137, 138, 139, 140, 141, 142, 143, 144, 145, 146, 147, 148, 149, 150, 151, 152, 153, 154, 155, 156, 157, 158, 159, 160, 161, 162, 163, 164, 165, 166, 167, 168, 169, 170, 171, 172, 173, 174, 175, 176, 177, 178, 179, 180, 181, 182, 183, 184, 185, 186, 187, 188, 189, 190, 191, 192, 193, 194, 195, 196, 197, 198, 199, 200, 201, 202, 203, 204, 205, 206, 207, 208, 209, 210, 211, 212, 213, 214, 215, 216, 217, 218, 219, 220, 221, 222, 223, 224, 225, 226, 227, 228, 229, 230, 231, 232, 233, 234, 235, 236, 237, 238, 239, 240, 241, 242, 243, 244, 245, 246, 247, 248, 249, 250, 251, 252, 253, 254, 255, 256, 257, 258, 259, 260, 261, 262, 263, 264, 265, 266, 267, 268, 269, 270, 271, 272, 273, 274, 275, 276, 277, 278, 279, 280, 281, 282, 283, 284, 285, 286, 287, 288, 289, 290, 291, 292, 293, 294, 295, 296, 297, 298, 299], "data y"=[2040, 2043, 2075, 2050, 2048, 2061, 2067, 2062, 2037, 2048, 2045, 2026, 2052, 2086, 2044, 2045, 2071, 2051, 2066, 2059, 2051, 2053, 2040, 2072, 2077, 2071, 2082, 2067, 2054, 2067, 2065, 2056, 2056, 2053, 2067, 2066, 2048, 2064, 2047, 2047, 2086, 2056, 2050, 2076, 2050, 2063, 2050, 2062, 2066, 2038, 2066, 2069, 2049, 2058, 2073, 2064, 2045, 2075, 2070, 2052, 2056, 2066, 2048, 2048, 2084, 2071, 2024, 2035, 2056, 2068, 2079, 2026, 2040, 2042, 2038, 2041, 2067, 2059, 2050, 2057, 2044, 2044, 2068, 2061, 2054, 2047, 2064, 2058, 2047, 2060, 2055, 2047, 2064, 2058, 2045, 2055, 2042, 2071, 2047, 2046, 2055, 2047, 2068, 2069, 2047, 2056, 2068, 2032, 2042, 2042, 2056, 2040, 2048, 2067, 2068, 2049, 2063, 2039, 2033, 2051, 2066, 2050, 2030, 2053, 2063, 2056, 2051, 2066, 2044, 2054, 2069, 2054, 2052, 2064, 2049, 2055, 2035, 2058, 2062, 2038, 2056, 2068, 2047, 2059, 2068, 2038, 2044, 2069, 2059, 2045, 2042, 2068, 2062, 2042, 2062, 2061, 2036, 2060, 2071, 2047, 2058, 2042, 2055, 2048, 2043, 2067, 2059, 2043, 2061, 2071, 2052, 2061, 2069, 2047, 2039, 2041, 2073, 2065, 2049, 2063, 2055, 2040, 2056, 2057, 2049, 2059, 2065, 2068, 2064, 2055, 2048, 2045, 2032, 2045, 2053, 2044, 2065, 2065, 2038, 2055, 2049, 2057, 2039, 2044, 2053, 2036, 2055, 2071, 2047, 2048, 2064, 2041, 2045, 2043, 2065, 2048, 2047, 2063, 2050, 2047, 2062, 2043, 2036, 2054, 2041, 2057, 2036, 2050, 2055, 2040, 2059, 2060, 2032, 2043, 2051, 2035, 2053, 2056, 2053, 2045, 2047, 2064, 2053, 2040, 2046, 2032, 2027, 2059, 2062, 2057, 2073, 2051, 2062, 2051, 2066, 2068, 2042, 2042, 2060, 2047, 2056, 2067, 2034, 2035, 2047, 2061, 2044, 2042, 2065, 2062, 2049, 2064, 2046, 2040, 2065, 2057, 2043, 2045, 2055, 2062, 2039, 2043, 2056, 2047, 2062, 2079, 2059, 2049, 2054, 2033, 2061, 2052, 2067, 2058, 2043, 2055, 2044, 2037, 2061, 2065]}, {"time"=[0, 1, 2, 3, 4, 5, 6, 7, 8, 9, 10, 11, 12, 13, 14, 15, 16, 17, 18, 19, 20, 21, 22, 23, 24, 25, 26, 27, 28, 29, 30, 31, 32, 33, 34, 35, 36, 37, 38, 39, 40, 41, 42, 43, 44, 45, 46, 47, 48, 49, 50, 51, 52, 53, 54, 55, 56, 57, 58, 59, 60, 61, 62, 63, 64, 65, 66, 67, 68, 69, 70, 71, 72, 73, 74, 75, 76, 77, 78, 79, 80, 81, 82, 83, 84, 85, 86, 87, 88, 89, 90, 91, 92, 93, 94, 95, 96, 97, 98, 99, 100, 101, 102, 103, 104, 105, 106, 107, 108, 109, 110, 111, 112, 113, 114, 115, 116, 117, 118, 119, 120, 121, 122, 123, 124, 125, 126, 127, 128, 129, 130, 131, 132, 133, 134, 135, 136, 137, 138, 139, 140, 141, 142, 143, 144, 145, 146, 147, 148, 149, 150, 151, 152, 153, 154, 155, 156, 157, 158, 159, 160, 161, 162, 163, 164, 165, 166, 167, 168, 169, 170, 171, 172, 173, 174, 175, 176, 177, 178, 179, 180, 181, 182, 183, 184, 185, 186, 187, 188, 189, 190, 191, 192, 193, 194, 195, 196, 197, 198, 199, 200, 201, 202, 203, 204, 205, 206, 207, 208, 209, 210, 211, 212, 213, 214, 215, 216, 217, 218, 219, 220, 221, 222, 223, 224, 225, 226, 227, 228, 229, 230, 231, 232, 233, 234, 235, 236, 237, 238, 239, 240, 241, 242, 243, 244, 245, 246, 247, 248, 249, 250, 251, 252, 253, 254, 255, 256, 257, 258, 259, 260, 261, 262, 263, 264, 265, 266, 267, 268, 269, 270, 271, 272, 273, 274, 275, 276, 277, 278, 279, 280, 281, 282, 283, 284, 285, 286, 287, 288, 289, 290, 291, 292, 293, 294, 295, 296, 297, 298, 299], "data y"=[2042, 2048, 2034, 2031, 2045, 2036, 2044, 2051, 2069, 2069, 2068, 2084, 2077, 2051, 2039, 2063, 2045, 2050, 2057, 2064, 2038, 2019, 2030, 2016, 2038, 2062, 2046, 2039, 2037, 2026, 2036, 2055, 2046, 2050, 2037, 2053, 2063, 2039, 2055, 2039, 2033, 2031, 2054, 2058, 2048, 2035, 2035, 2042, 2017, 2025, 2041, 2019, 2033, 2039, 2027, 2036, 2039, 2044, 2043, 2032, 2058, 2045, 2046, 2049, 2043, 2035, 2051, 2061, 2055, 2035, 2030, 2065, 2071, 2055, 2056, 2053, 2048, 2042, 2045, 2038, 2051, 2057, 2035, 2023, 2033, 2045, 2039, 2033, 2042, 2037, 2034, 2047, 2034, 2029, 2035, 2043, 2047, 2025, 2045, 2053, 2037, 2044, 2048, 2030, 2041, 2037, 2045, 2053, 2046, 2057, 2048, 2052, 2046, 2031, 2030, 2061, 2061, 2050, 2048, 2034, 2025, 2027, 2037, 2030, 2019, 2022, 2040, 2048, 2057, 2060, 2033, 2039, 2058, 2038, 2043, 2036, 2045, 2056, 2038, 2045, 2052, 2031, 2040, 2038, 2040, 2042, 2055, 2045, 2035, 2041, 2054, 2037, 2034, 2037, 2032, 2035, 2047, 2046, 2035, 2046, 2049, 2044, 2038, 2044, 2043, 2032, 2037, 2047, 2041, 2029, 2040, 2051, 2038, 2041, 2042, 2053, 2039, 2027, 2041, 2040, 2033, 2039, 2037, 2026, 2035, 2035, 2039, 2051, 2046, 2046, 2047, 2043, 2046, 2039, 2028, 2045, 2043, 2035, 2055, 2054, 2047, 2039, 2041, 2040, 2013, 2034, 2046, 2029, 2037, 2045, 2037, 2051, 2049, 2047, 2037, 2034, 2050, 2034, 2027, 2043, 2035, 2037, 2052, 2050, 2039, 2030, 2046, 2032, 2045, 2055, 2072, 2068, 2098, 2090, 2074, 2081, 2075, 2043, 2026, 2020, 2030, 2031, 2030, 2043, 2032, 2022, 2026, 2022, 2023, 2024, 2013, 2021, 2029, 2041, 2030, 2031, 2038, 2031, 2024, 2032, 2039, 2041, 2060, 2059, 2044, 2029, 2033, 2050, 2037, 2031, 2034, 2035, 2040, 2046, 2043, 2043, 2051, 2047, 2043, 2036, 2041, 2054, 2054, 2047, 2056, 2045, 2043, 2039, 2037, 2050, 2026, 2042, 2036, 2024, 2044, 2045, 2035, 2044, 2039, 2041]}]
  out "max/min x5":bool
  out "max/min y5":bool
  out "deviation error x5":bool
  out "deviation error y5":bool
  out "error x5":bool
  out "error y5":bool
  out "deviation y5":dbl=19225.96412953808
  out "deviation x5":dbl=12582043.816128
  out "min y5 now":i16=2002
  out "min x5 now":i16=621
  out "max x5 now":i16=2672
  out "max y5 now":i16=2101
  out "template max x5":i16=2672
  out "template min x5":i16=621
  out "template min y5":i16=2013
  out "template max y5":i16=2098
  out "size now":i32=300
  out "template size":i32=300
  out "template min x3":i16=1604
  out "template max x3":i16=2080
  out "template min y3":i16=2024
  out "template max y3":i16=2086
  out "max x3 now":i16=2081
  out "min x3 now":i16=1624
  out "max y3 now":i16=2087
  out "min y3 now":i16=2024
  out "deviation x3":dbl=362328.184763864
  out "deviation y3":dbl=15488.579850463302
  out "deviation y3 min":dbl=254.46333333333362
  out "deviation x3 min":dbl=458.2599999999992
  out "deviation y5 min":dbl=186.01000000000005
  out "deviation x5 min":dbl=377.9399999999985
  in  "gathered err x 3":i16[](array[numeric])=[1986, 1970, 1920, 1858, 1861, 1860, 1808, 1774, 1734, 1748, 1695, 1675, 1665, 1650, 1668, 1624, 1652, 1624, 1636, 1627, 1647, 1655, 1677, 1675, 1696, 1728, 1732, 1725, 1767, 1796, 1796, 1846, 1885, 1873, 1909, 1930, 1975, 1952, 1993, 2008, 2014, 1986, 2017, 2037, 2018, 2020, 2017, 1998, 1997, 2030, 2037, 2018, 2013, 2029, 2019, 2007, 2043, 2014, 2019, 2007, 2050, 2067, 1998, 1985, 2043, 2057, 2007, 1991, 1987, 2004, 2037, 2047, 2025, 2039, 2020, 2050, 2026, 2017, 2027, 1996, 1995, 2047, 2055, 2019, 2007, 2022, 2029, 1994, 2029, 2067, 2028, 2005, 2024, 2042, 2033, 2047, 2027, 2005, 2016, 2041, 2018, 2017, 2008, 2015, 2025, 2052, 2056, 2042, 2049, 2011, 2005, 2043, 2052, 2027, 2021, 2058, 2051, 2038, 2045, 2022, 2015, 2048, 2058, 2047, 2061, 2024, 2039, 2035, 2055, 2055, 2022, 2037, 2039, 2014, 2036, 2053, 2025, 2054, 2042, 2058, 2034, 2044, 2063, 2042, 2023, 2043, 2027, 2039, 2067, 2063, 2047, 2011, 2045, 2057, 2037, 2051, 2049, 2016, 2038, 2064, 2038, 2041, 2053, 2027, 2045, 2040, 2064, 2037, 2020, 2047, 2047, 2032, 2068, 2049, 2023, 2035, 2043, 2081, 2038, 2041, 2045, 2010, 2028, 2059, 2045, 2050, 2067, 2035, 2035, 2059, 2051, 2040, 2025, 2051, 2052, 2031, 2063, 2062, 2027, 2051, 2054, 2022, 2036, 2040, 2057, 2037, 2048, 2064, 2038, 2033, 2058, 2045, 2037, 2051, 2027, 2053, 2025, 2031, 2033, 2023, 2049, 2053, 2038, 2054, 2050, 2025, 2041, 2067, 2039, 2016, 2030, 2056, 2045, 2052, 2067, 2029, 2027, 2045, 2023, 2031, 2065, 2065, 2053, 2041, 2057, 2037, 2017, 2027, 2027, 2028, 2064, 2078, 2042, 2045, 2036, 2069, 2043, 2032, 2038, 2018, 2047, 2072, 2041, 2045, 2053, 2026, 2030, 2016, 2034, 2023, 2025, 2065, 2047, 2029, 2041, 2029, 2032, 2067, 2054, 2031, 2051, 2067, 2051, 2016, 2036, 2063, 2047, 2060, 2064, 2026, 2024, 2045, 2026, 2028, 2012, 2034, 2026, 2031, 2055, 2041]
  in  "gathered err y 3":i16[](array[numeric])=[2052, 2061, 2063, 2041, 2035, 2058, 2066, 2066, 2068, 2062, 2054, 2045, 2073, 2074, 2031, 2080, 2051, 2055, 2053, 2054, 2043, 2050, 2071, 2049, 2039, 2046, 2056, 2052, 2059, 2073, 2060, 2061, 2059, 2053, 2058, 2041, 2063, 2064, 2041, 2074, 2068, 2060, 2061, 2064, 2053, 2064, 2069, 2050, 2057, 2054, 2058, 2068, 2050, 2066, 2058, 2050, 2048, 2081, 2035, 2068, 2067, 2055, 2041, 2070, 2087, 2039, 2024, 2054, 2084, 2074, 2072, 2075, 2054, 2050, 2042, 2059, 2070, 2058, 2070, 2066, 2030, 2041, 2074, 2068, 2051, 2046, 2038, 2042, 2033, 2063, 2075, 2051, 2043, 2045, 2055, 2072, 2070, 2055, 2048, 2075, 2054, 2057, 2058, 2055, 2044, 2046, 2064, 2059, 2068, 2056, 2038, 2052, 2062, 2062, 2038, 2053, 2076, 2054, 2060, 2063, 2037, 2046, 2061, 2046, 2058, 2035, 2053, 2046, 2052, 2063, 2052, 2047, 2059, 2040, 2038, 2060, 2050, 2050, 2053, 2059, 2052, 2039, 2063, 2065, 2052, 2055, 2054, 2039, 2056, 2066, 2056, 2029, 2034, 2060, 2058, 2056, 2072, 2053, 2039, 2055, 2052, 2045, 2060, 2057, 2065, 2049, 2063, 2074, 2046, 2047, 2055, 2032, 2047, 2072, 2051, 2051, 2066, 2072, 2070, 2051, 2059, 2046, 2032, 2047, 2057, 2052, 2073, 2073, 2049, 2057, 2053, 2063, 2048, 2046, 2064, 2046, 2057, 2075, 2056, 2049, 2067, 2045, 2041, 2046, 2059, 2061, 2046, 2060, 2055, 2037, 2051, 2062, 2055, 2063, 2060, 2080, 2051, 2046, 2047, 2029, 2038, 2060, 2054, 2060, 2074, 2052, 2047, 2053, 2057, 2048, 2032, 2054, 2054, 2047, 2064, 2059, 2037, 2043, 2051, 2044, 2065, 2045, 2059, 2050, 2065, 2071, 2047, 2042, 2047, 2033, 2042, 2064, 2058, 2053, 2031, 2065, 2064, 2049, 2059, 2047, 2044, 2053, 2059, 2053, 2069, 2059, 2033, 2041, 2045, 2053, 2035, 2046, 2064, 2045, 2051, 2058, 2041, 2052, 2068, 2054, 2055, 2060, 2071, 2055, 2038, 2060, 2052, 2047, 2069, 2058, 2042, 2056, 2049, 2066, 2040, 2050, 2056, 2034, 2055, 2059]
  in  "template err x 3":i16[](array[numeric])=[1987, 1971, 1955, 1885, 1866, 1853, 1810, 1748, 1734, 1732, 1693, 1670, 1650, 1620, 1668, 1631, 1633, 1604, 1653, 1636, 1640, 1666, 1683, 1678, 1678, 1708, 1728, 1718, 1749, 1797, 1795, 1816, 1846, 1904, 1919, 1903, 1949, 1977, 1957, 2028, 2013, 1998, 2012, 2026, 2009, 2022, 2026, 2052, 2031, 2007, 2043, 2018, 2015, 2033, 2040, 1992, 2027, 2023, 2033, 2030, 1985, 2043, 2038, 1979, 2014, 2055, 2048, 2007, 1978, 1979, 2011, 1998, 2018, 2016, 2008, 2028, 2038, 2005, 2018, 2031, 2005, 2038, 2052, 2009, 2023, 2027, 2046, 2020, 2020, 2044, 2019, 2027, 2049, 2016, 2006, 2046, 2025, 2014, 2006, 2032, 2035, 2051, 2066, 2024, 2004, 2035, 2037, 2024, 2053, 2028, 2035, 2032, 2053, 2061, 2024, 2034, 2050, 2011, 2030, 2053, 2036, 2023, 2037, 2053, 2038, 2015, 2038, 2049, 2038, 2057, 2054, 2015, 2040, 2055, 2035, 2017, 2023, 2059, 2050, 2052, 2074, 2039, 2027, 2049, 2031, 2026, 2058, 2069, 2056, 2031, 2058, 2069, 2027, 2018, 2049, 2031, 2034, 2067, 2053, 2042, 2059, 2039, 2051, 2027, 2047, 2065, 2031, 2036, 2064, 2048, 2042, 2060, 2048, 2026, 2027, 2058, 2069, 2034, 2041, 2059, 2032, 2054, 2071, 2037, 2035, 2032, 2034, 2065, 2038, 2032, 2036, 2027, 2025, 2055, 2029, 2029, 2058, 2039, 2033, 2063, 2047, 2035, 2014, 2039, 2033, 2022, 2058, 2042, 2024, 2053, 2049, 2027, 2053, 2041, 2041, 2021, 2048, 2055, 2028, 2045, 2047, 2020, 2031, 2042, 2020, 2027, 2034, 2057, 2036, 2044, 2065, 2026, 2014, 2035, 2030, 2024, 2058, 2040, 2042, 2025, 2048, 2055, 2032, 2042, 2053, 2024, 2042, 2072, 2053, 2054, 2054, 2066, 2045, 2045, 2063, 2039, 2026, 2044, 2030, 2020, 2052, 2039, 2019, 2053, 2034, 2046, 2022, 2057, 2077, 2044, 2045, 2048, 2019, 2031, 2049, 2026, 2027, 2032, 2049, 2029, 2009, 2046, 2052, 2051, 2080, 2061, 2033, 2040, 2029, 2012, 2032, 2044, 2065, 2034, 2037, 2056, 2031, 2042, 2072, 2046]
  in  "template err y 3":i16[](array[numeric])=[2040, 2043, 2075, 2050, 2048, 2061, 2067, 2062, 2037, 2048, 2045, 2026, 2052, 2086, 2044, 2045, 2071, 2051, 2066, 2059, 2051, 2053, 2040, 2072, 2077, 2071, 2082, 2067, 2054, 2067, 2065, 2056, 2056, 2053, 2067, 2066, 2048, 2064, 2047, 2047, 2086, 2056, 2050, 2076, 2050, 2063, 2050, 2062, 2066, 2038, 2066, 2069, 2049, 2058, 2073, 2064, 2045, 2075, 2070, 2052, 2056, 2066, 2048, 2048, 2084, 2071, 2024, 2035, 2056, 2068, 2079, 2026, 2040, 2042, 2038, 2041, 2067, 2059, 2050, 2057, 2044, 2044, 2068, 2061, 2054, 2047, 2064, 2058, 2047, 2060, 2055, 2047, 2064, 2058, 2045, 2055, 2042, 2071, 2047, 2046, 2055, 2047, 2068, 2069, 2047, 2056, 2068, 2032, 2042, 2042, 2056, 2040, 2048, 2067, 2068, 2049, 2063, 2039, 2033, 2051, 2066, 2050, 2030, 2053, 2063, 2056, 2051, 2066, 2044, 2054, 2069, 2054, 2052, 2064, 2049, 2055, 2035, 2058, 2062, 2038, 2056, 2068, 2047, 2059, 2068, 2038, 2044, 2069, 2059, 2045, 2042, 2068, 2062, 2042, 2062, 2061, 2036, 2060, 2071, 2047, 2058, 2042, 2055, 2048, 2043, 2067, 2059, 2043, 2061, 2071, 2052, 2061, 2069, 2047, 2039, 2041, 2073, 2065, 2049, 2063, 2055, 2040, 2056, 2057, 2049, 2059, 2065, 2068, 2064, 2055, 2048, 2045, 2032, 2045, 2053, 2044, 2065, 2065, 2038, 2055, 2049, 2057, 2039, 2044, 2053, 2036, 2055, 2071, 2047, 2048, 2064, 2041, 2045, 2043, 2065, 2048, 2047, 2063, 2050, 2047, 2062, 2043, 2036, 2054, 2041, 2057, 2036, 2050, 2055, 2040, 2059, 2060, 2032, 2043, 2051, 2035, 2053, 2056, 2053, 2045, 2047, 2064, 2053, 2040, 2046, 2032, 2027, 2059, 2062, 2057, 2073, 2051, 2062, 2051, 2066, 2068, 2042, 2042, 2060, 2047, 2056, 2067, 2034, 2035, 2047, 2061, 2044, 2042, 2065, 2062, 2049, 2064, 2046, 2040, 2065, 2057, 2043, 2045, 2055, 2062, 2039, 2043, 2056, 2047, 2062, 2079, 2059, 2049, 2054, 2033, 2061, 2052, 2067, 2058, 2043, 2055, 2044, 2037, 2061, 2065]
  in  "time":i32[](array[numeric])=[0, 1, 2, 3, 4, 5, 6, 7, 8, 9, 10, 11, 12, 13, 14, 15, 16, 17, 18, 19, 20, 21, 22, 23, 24, 25, 26, 27, 28, 29, 30, 31, 32, 33, 34, 35, 36, 37, 38, 39, 40, 41, 42, 43, 44, 45, 46, 47, 48, 49, 50, 51, 52, 53, 54, 55, 56, 57, 58, 59, 60, 61, 62, 63, 64, 65, 66, 67, 68, 69, 70, 71, 72, 73, 74, 75, 76, 77, 78, 79, 80, 81, 82, 83, 84, 85, 86, 87, 88, 89, 90, 91, 92, 93, 94, 95, 96, 97, 98, 99, 100, 101, 102, 103, 104, 105, 106, 107, 108, 109, 110, 111, 112, 113, 114, 115, 116, 117, 118, 119, 120, 121, 122, 123, 124, 125, 126, 127, 128, 129, 130, 131, 132, 133, 134, 135, 136, 137, 138, 139, 140, 141, 142, 143, 144, 145, 146, 147, 148, 149, 150, 151, 152, 153, 154, 155, 156, 157, 158, 159, 160, 161, 162, 163, 164, 165, 166, 167, 168, 169, 170, 171, 172, 173, 174, 175, 176, 177, 178, 179, 180, 181, 182, 183, 184, 185, 186, 187, 188, 189, 190, 191, 192, 193, 194, 195, 196, 197, 198, 199, 200, 201, 202, 203, 204, 205, 206, 207, 208, 209, 210, 211, 212, 213, 214, 215, 216, 217, 218, 219, 220, 221, 222, 223, 224, 225, 226, 227, 228, 229, 230, 231, 232, 233, 234, 235, 236, 237, 238, 239, 240, 241, 242, 243, 244, 245, 246, 247, 248, 249, 250, 251, 252, 253, 254, 255, 256, 257, 258, 259, 260, 261, 262, 263, 264, 265, 266, 267, 268, 269, 270, 271, 272, 273, 274, 275, 276, 277, 278, 279, 280, 281, 282, 283, 284, 285, 286, 287, 288, 289, 290, 291, 292, 293, 294, 295, 296, 297, 298, 299]
  out "error x 5 now":i16[](array[numeric])=[2031, 2054, 2044, 2020, 2028, 2026, 2038, 2032, 2038, 2052, 2051, 2045, 2052, 2046, 2035, 2047, 2043, 2036, 2028, 2038, 2051, 2042, 2033, 2029, 2035, 2043, 2060, 2055, 2033, 2037, 2044, 2041, 2039, 2042, 2048, 2039, 2050, 2042, 2030, 2039, 2042, 2034, 2037, 2048, 2059, 2039, 2035, 2035, 2032, 2041, 2051, 2038, 2036, 2039, 2045, 2042, 2042, 2049, 2028, 2031, 2036, 2041, 2048, 2056, 2048, 2025, 2034, 2037, 2026, 2042, 2045, 2058, 2040, 2028, 2043, 2033, 2039, 2064, 2056, 2046, 2052, 2042, 2039, 2027, 2041, 2048, 2036, 2049, 2056, 2047, 2047, 2043, 2028, 2039, 2046, 2058, 2039, 2033, 2035, 2035, 2033, 2043, 2035, 2040, 2053, 2050, 2049, 2045, 2044, 2051, 2030, 2038, 2051, 2038, 2047, 2050, 2040, 2047, 2055, 2033, 2055, 2049, 2049, 2041, 2033, 2045, 2042, 2033, 2050, 2058, 2042, 2049, 2050, 2049, 2036, 2041, 2047, 2039, 2041, 2053, 2036, 2043, 2053, 2048, 2040, 2050, 2049, 2055, 2042, 2037]
  out "error y 5 now":i16[](array[numeric])=[2036, 2036, 2036, 2027, 2041, 2049, 2053, 2045, 2033, 2036, 2043, 2038, 2041, 2048, 2028, 2040, 2061, 2051, 2042, 2027, 2042, 2055, 2032, 2026, 2042, 2037, 2044, 2064, 2046, 2027, 2053, 2049, 2046, 2037, 2047, 2043, 2044, 2047, 2049, 2045, 2040, 2031, 2039, 2038, 2048, 2055, 2031, 2025, 2025, 2033, 2046, 2051, 2054, 2062, 2044, 2036, 2035, 2046, 2045, 2033, 2038, 2042, 2047, 2053, 2058, 2046, 2052, 2052, 2037, 2051, 2037, 2042, 2043, 2029, 2034, 2039, 2029, 2043, 2049, 2048, 2050, 2035, 2049, 2049, 2043, 2046, 2036, 2040, 2042, 2032, 2033, 2056, 2049, 2019, 2046, 2056, 2058, 2047, 2045, 2045, 2034, 2038, 2048, 2050, 2056, 2054, 2032, 2033, 2038, 2040, 2045, 2035, 2051, 2045, 2031, 2038, 2045, 2042, 2048, 2050, 2057, 2042, 2040, 2054, 2042, 2031, 2038, 2040, 2030, 2051, 2047, 2044, 2060, 2046, 2035, 2026, 2044, 2039, 2042, 2048, 2059, 2053, 2042, 2047, 2051, 2047, 2029, 2049, 2046, 2037]
  out "error y 3 now":i16[](array[numeric])=[2068, 2051, 2035, 2052, 2049, 2060, 2029, 2046, 2069, 2056, 2055, 2055, 2034, 2045, 2070, 2055, 2046, 2047, 2067, 2061, 2039, 2034, 2051, 2048, 2059, 2067, 2047, 2037, 2058, 2053, 2044, 2042, 2066, 2060, 2043, 2052, 2037, 2041, 2051, 2043, 2030, 2050, 2044, 2054, 2036, 2047, 2055, 2042, 2056, 2057, 2036, 2045, 2054, 2043, 2057, 2072, 2051, 2030, 2044, 2068, 2059, 2056, 2065, 2042, 2029, 2050, 2042, 2040, 2065, 2054, 2061, 2038, 2053, 2055, 2032, 2055, 2061, 2039, 2046, 2053, 2030, 2036, 2029, 2049, 2043, 2052, 2074, 2061, 2048, 2058, 2043, 2028, 2047, 2053, 2057, 2039, 2049, 2063, 2043, 2056, 2063, 2047, 2046, 2059, 2049, 2050, 2059, 2060, 2049, 2034, 2049, 2053, 2047, 2070, 2063, 2039, 2041, 2042, 2025, 2049, 2052, 2060, 2032, 2037, 2059, 2052, 2039, 2062, 2048, 2041, 2066, 2056, 2037, 2038, 2052, 2060, 2035, 2053, 2072, 2053, 2060, 2068, 2041, 2035, 2049, 2037, 2055, 2034, 2042, 2055]
  in  "reset":i16[](array[numeric])
  in  "gathered err x 5":i16[](array[numeric])=[2382, 2659, 2664, 2672, 2666, 2654, 2660, 2664, 2667, 2655, 2663, 2668, 2662, 2667, 2660, 2658, 2661, 2670, 2657, 2659, 2671, 2214, 1624, 1315, 1097, 961, 861, 782, 703, 622, 628, 628, 621, 632, 635, 636, 668, 754, 892, 1012, 1172, 1362, 1513, 1661, 1801, 1899, 1955, 2029, 2076, 2101, 2109, 2111, 2110, 2082, 2059, 2050, 2019, 2037, 2053, 2067, 2089, 2092, 2091, 2116, 2097, 2066, 2077, 2087, 2092, 2091, 2075, 2066, 2058, 2046, 2042, 2030, 2048, 2065, 2051, 2053, 2073, 2052, 2041, 2052, 2058, 2057, 2062, 2070, 2067, 2039, 2044, 2048, 2041, 2035, 2026, 2037, 2059, 2060, 2064, 2055, 2051, 2045, 2046, 2067, 2066, 2040, 2041, 2052, 2045, 2056, 2059, 2044, 2042, 2049, 2042, 2045, 2048, 2064, 2060, 2052, 2064, 2055, 2049, 2055, 2038, 2049, 2038, 2059, 2059, 2059, 2053, 2052, 2046, 2056, 2051, 2029, 2043, 2048, 2054, 2041, 2058, 2056, 2039, 2045, 2065, 2054, 2055, 2056, 2040, 2049, 2055, 2052, 2042, 2044, 2058, 2064, 2055, 2068, 2065, 2050, 2052, 2058, 2039, 2040, 2037, 2050, 2054, 2060, 2067, 2043, 2053, 2057, 2047, 2037, 2050, 2054, 2047, 2035, 2047, 2063, 2052, 2061, 2064, 2047, 2055, 2066, 2056, 2062, 2068, 2061, 2042, 2035, 2047, 2037, 2034, 2043, 2046, 2039, 2053, 2058, 2051, 2070, 2063, 2056, 2042, 2055, 2069, 2039, 2044, 2052, 2049, 2048, 2061, 2059, 2057, 2043, 2058, 2052, 2041, 2054, 2044, 2038, 2048, 2045, 2043, 2072, 2072, 2057, 2058, 2056, 2063, 2049, 2054, 2056, 2047, 2046, 2059, 2041, 2042, 2055, 2052, 2045, 2045, 2059, 2050, 2057, 2068, 2054, 2051, 2057, 2041, 2031, 2051, 2048, 2056, 2040, 2050, 2056, 2045, 2062, 2059, 2035, 2032, 2053, 2042, 2056, 2063, 2063, 2048, 2052, 2065, 2057, 2044, 2053, 2053, 2043, 2050, 2058, 2035, 2058, 2049, 2058, 2047, 2056, 2061, 2045, 2052, 2054, 2042, 2051, 2051, 2056, 2062, 2047, 2066, 2048, 2050, 2062, 2056, 2049]
  in  "gathered err y 5":i16[](array[numeric])=[2038, 2035, 2029, 2040, 2046, 2033, 2032, 2044, 2045, 2051, 2047, 2071, 2062, 2041, 2051, 2057, 2045, 2056, 2044, 2031, 2045, 2055, 2077, 2043, 2027, 2024, 2008, 2031, 2040, 2035, 2041, 2047, 2038, 2036, 2058, 2071, 2043, 2042, 2051, 2057, 2038, 2058, 2064, 2032, 2042, 2053, 2038, 2035, 2028, 2043, 2031, 2041, 2046, 2044, 2028, 2042, 2034, 2027, 2025, 2040, 2014, 2026, 2051, 2058, 2041, 2044, 2072, 2066, 2044, 2037, 2040, 2038, 2050, 2052, 2053, 2048, 2038, 2045, 2049, 2031, 2056, 2055, 2035, 2034, 2051, 2053, 2052, 2037, 2060, 2043, 2027, 2029, 2040, 2037, 2028, 2041, 2035, 2024, 2049, 2039, 2034, 2036, 2030, 2050, 2050, 2042, 2036, 2041, 2036, 2038, 2041, 2030, 2043, 2044, 2053, 2056, 2047, 2055, 2049, 2029, 2034, 2048, 2041, 2044, 2050, 2044, 2036, 2047, 2050, 2022, 2023, 2032, 2040, 2034, 2051, 2043, 2039, 2044, 2052, 2049, 2040, 2048, 2033, 2021, 2034, 2032, 2026, 2049, 2051, 2034, 2049, 2054, 2055, 2045, 2049, 2058, 2048, 2048, 2057, 2047, 2044, 2046, 2037, 2032, 2044, 2043, 2042, 2032, 2034, 2048, 2045, 2053, 2054, 2031, 2015, 2032, 2032, 2030, 2030, 2033, 2039, 2045, 2062, 2048, 2044, 2052, 2047, 2027, 2037, 2043, 2049, 2047, 2051, 2046, 2033, 2036, 2036, 2037, 2042, 2055, 2035, 2032, 2038, 2037, 2035, 2038, 2060, 2053, 2043, 2046, 2047, 2045, 2048, 2042, 2041, 2026, 2028, 2049, 2045, 2045, 2052, 2041, 2038, 2036, 2027, 2029, 2047, 2045, 2034, 2051, 2081, 2094, 2083, 2101, 2093, 2078, 2070, 2061, 2036, 2027, 2027, 2036, 2012, 2002, 2022, 2018, 2024, 2027, 2021, 2021, 2036, 2025, 2035, 2036, 2026, 2039, 2024, 2029, 2031, 2039, 2062, 2048, 2038, 2039, 2042, 2041, 2055, 2036, 2039, 2029, 2045, 2055, 2034, 2033, 2041, 2037, 2056, 2052, 2037, 2027, 2027, 2038, 2036, 2038, 2050, 2061, 2054, 2046, 2028, 2029, 2036, 2040, 2034, 2027, 2028, 2037, 2025, 2050, 2048, 2041]
  in  "num of elem array":i32[](array[numeric])=[0, 1, 2, 3, 4, 5, 6, 7, 8, 9, 10, 11, 12, 13, 14, 15, 16, 17, 18, 19, 20, 21, 22, 23, 24, 25, 26, 27, 28, 29, 30, 31, 32, 33, 34, 35, 36, 37, 38, 39, 40, 41, 42, 43, 44, 45, 46, 47, 48, 49, 50, 51, 52, 53, 54, 55, 56, 57, 58, 59, 60, 61, 62, 63, 64, 65, 66, 67, 68, 69, 70, 71, 72, 73, 74, 75, 76, 77, 78, 79, 80, 81, 82, 83, 84, 85, 86, 87, 88, 89, 90, 91, 92, 93, 94, 95, 96, 97, 98, 99, 100, 101, 102, 103, 104, 105, 106, 107, 108, 109, 110, 111, 112, 113, 114, 115, 116, 117, 118, 119, 120, 121, 122, 123, 124, 125, 126, 127, 128, 129, 130, 131, 132, 133, 134, 135, 136, 137, 138, 139, 140, 141, 142, 143, 144, 145, 146, 147, 148, 149]
  out "error x 3 now":i16[](array[numeric])=[2071, 2039, 2036, 2051, 2051, 2040, 2029, 2062, 2055, 2035, 2053, 2044, 2025, 2060, 2073, 2030, 2042, 2039, 2050, 2027, 2018, 2046, 2065, 2037, 2057, 2053, 2030, 2049, 2072, 2034, 2032, 2069, 2083, 2035, 2030, 2040, 2024, 2055, 2070, 2033, 2041, 2049, 2031, 2029, 2032, 2062, 2045, 2038, 2054, 2026, 2016, 2048, 2049, 2056, 2084, 2060, 2040, 2028, 2066, 2074, 2043, 2052, 2055, 2015, 2037, 2057, 2029, 2048, 2069, 2071, 2045, 2044, 2061, 2031, 2028, 2050, 2031, 2019, 2047, 2042, 2042, 2005, 2029, 2053, 2044, 2072, 2074, 2039, 2044, 2049, 2016, 2032, 2063, 2045, 2044, 2043, 2073, 2063, 2043, 2058, 2045, 2025, 2047, 2057, 2042, 2063, 2066, 2051, 2019, 2033, 2062, 2055, 2062, 2069, 2033, 2017, 2035, 2015, 2027, 2069, 2055, 2051, 2026, 2055, 2066, 2026, 2042, 2049, 2025, 2052, 2074, 2037, 2052, 2032, 2052, 2038, 2035, 2071, 2063, 2047, 2063, 2041, 2011, 2026, 2048, 2036, 2023, 2027, 2061, 2046]
  in  "template err y 5":i16[](array[numeric])=[2042, 2048, 2034, 2031, 2045, 2036, 2044, 2051, 2069, 2069, 2068, 2084, 2077, 2051, 2039, 2063, 2045, 2050, 2057, 2064, 2038, 2019, 2030, 2016, 2038, 2062, 2046, 2039, 2037, 2026, 2036, 2055, 2046, 2050, 2037, 2053, 2063, 2039, 2055, 2039, 2033, 2031, 2054, 2058, 2048, 2035, 2035, 2042, 2017, 2025, 2041, 2019, 2033, 2039, 2027, 2036, 2039, 2044, 2043, 2032, 2058, 2045, 2046, 2049, 2043, 2035, 2051, 2061, 2055, 2035, 2030, 2065, 2071, 2055, 2056, 2053, 2048, 2042, 2045, 2038, 2051, 2057, 2035, 2023, 2033, 2045, 2039, 2033, 2042, 2037, 2034, 2047, 2034, 2029, 2035, 2043, 2047, 2025, 2045, 2053, 2037, 2044, 2048, 2030, 2041, 2037, 2045, 2053, 2046, 2057, 2048, 2052, 2046, 2031, 2030, 2061, 2061, 2050, 2048, 2034, 2025, 2027, 2037, 2030, 2019, 2022, 2040, 2048, 2057, 2060, 2033, 2039, 2058, 2038, 2043, 2036, 2045, 2056, 2038, 2045, 2052, 2031, 2040, 2038, 2040, 2042, 2055, 2045, 2035, 2041, 2054, 2037, 2034, 2037, 2032, 2035, 2047, 2046, 2035, 2046, 2049, 2044, 2038, 2044, 2043, 2032, 2037, 2047, 2041, 2029, 2040, 2051, 2038, 2041, 2042, 2053, 2039, 2027, 2041, 2040, 2033, 2039, 2037, 2026, 2035, 2035, 2039, 2051, 2046, 2046, 2047, 2043, 2046, 2039, 2028, 2045, 2043, 2035, 2055, 2054, 2047, 2039, 2041, 2040, 2013, 2034, 2046, 2029, 2037, 2045, 2037, 2051, 2049, 2047, 2037, 2034, 2050, 2034, 2027, 2043, 2035, 2037, 2052, 2050, 2039, 2030, 2046, 2032, 2045, 2055, 2072, 2068, 2098, 2090, 2074, 2081, 2075, 2043, 2026, 2020, 2030, 2031, 2030, 2043, 2032, 2022, 2026, 2022, 2023, 2024, 2013, 2021, 2029, 2041, 2030, 2031, 2038, 2031, 2024, 2032, 2039, 2041, 2060, 2059, 2044, 2029, 2033, 2050, 2037, 2031, 2034, 2035, 2040, 2046, 2043, 2043, 2051, 2047, 2043, 2036, 2041, 2054, 2054, 2047, 2056, 2045, 2043, 2039, 2037, 2050, 2026, 2042, 2036, 2024, 2044, 2045, 2035, 2044, 2039, 2041]
  in  "template err x 5":i16[](array[numeric])=[2274, 2661, 2656, 2670, 2664, 2659, 2660, 2663, 2671, 2660, 2661, 2665, 2662, 2671, 2670, 2652, 2672, 2662, 2664, 2661, 2536, 2114, 1733, 1378, 1144, 991, 891, 826, 740, 646, 631, 634, 626, 621, 629, 644, 660, 754, 876, 1004, 1154, 1319, 1494, 1608, 1738, 1913, 1993, 2036, 2074, 2107, 2096, 2091, 2094, 2073, 2052, 2044, 2041, 2029, 2058, 2070, 2099, 2101, 2082, 2103, 2102, 2076, 2063, 2070, 2099, 2107, 2095, 2067, 2066, 2055, 2044, 2046, 2042, 2063, 2063, 2042, 2058, 2045, 2047, 2048, 2053, 2065, 2056, 2055, 2059, 2040, 2053, 2049, 2035, 2046, 2051, 2052, 2047, 2037, 2062, 2057, 2043, 2051, 2043, 2052, 2058, 2049, 2055, 2056, 2044, 2047, 2039, 2056, 2042, 2033, 2052, 2065, 2051, 2055, 2064, 2046, 2044, 2050, 2062, 2041, 2041, 2060, 2054, 2045, 2065, 2043, 2034, 2051, 2056, 2051, 2068, 2050, 2045, 2038, 2047, 2056, 2041, 2045, 2057, 2052, 2059, 2059, 2052, 2043, 2058, 2068, 2062, 2051, 2045, 2061, 2044, 2050, 2055, 2048, 2047, 2054, 2043, 2050, 2040, 2044, 2045, 2046, 2052, 2060, 2051, 2045, 2055, 2047, 2056, 2071, 2049, 2052, 2049, 2062, 2063, 2064, 2065, 2067, 2041, 2046, 2048, 2033, 2044, 2032, 2052, 2057, 2060, 2049, 2053, 2039, 2046, 2056, 2045, 2052, 2060, 2059, 2042, 2042, 2049, 2045, 2043, 2055, 2054, 2053, 2065, 2056, 2054, 2061, 2047, 2055, 2042, 2059, 2051, 2037, 2046, 2054, 2049, 2059, 2056, 2039, 2040, 2048, 2058, 2055, 2062, 2066, 2046, 2057, 2069, 2056, 2041, 2046, 2040, 2037, 2043, 2059, 2050, 2042, 2049, 2057, 2052, 2046, 2038, 2030, 2043, 2066, 2054, 2046, 2051, 2060, 2041, 2046, 2053, 2056, 2047, 2051, 2052, 2048, 2065, 2057, 2066, 2045, 2048, 2060, 2047, 2052, 2069, 2054, 2057, 2066, 2042, 2051, 2057, 2053, 2040, 2040, 2048, 2053, 2040, 2046, 2049, 2048, 2068, 2064, 2065, 2055, 2060, 2063, 2048, 2057, 2054, 2046, 2061, 2042, 2022, 2044]
  out "Warning":string="must be greater than number of elements"
  in  "number of pts after trigger stops":i32=300
  out "end trigger":bool=TRUE
  in  "trigger treshold":i16=150
  out "trigger index":i32=149
  out "end trigger index":i32=122
  in  "x5 0 level":i16=2050
  in  "y5 0 level":i16=2050
  in  "Filename template":path=path "C:/Users/User/Desktop/Tester_znakowarki/generator_template/template.lvm" caption="Filename"
  in  "Filename errors":path=path "C:/Users/User/Desktop/Tester_znakowarki/generator_errors/error.lvm" caption="Filename"
  in  "Filename history":path=path "C:/Users/User/Desktop/Tester_znakowarki/generator_history/history.lvm" caption="Filename"
  in  "min/max precision err y 3":i16=30
  in  "min/max precision err y 5":i16=50
  in  "deviation precision err y 3":dbl=2000.0
  in  "deviation precision err y 5":dbl=6000.0
  in  "deviation precision err x 3":dbl=2000.0
  in  "min/max precision err x 3":i16=30
  in  "min/max precision err x 5":i16=50
  in  "deviation precision err x 5":dbl=6000.0
  out "trigger index 2":i32=122
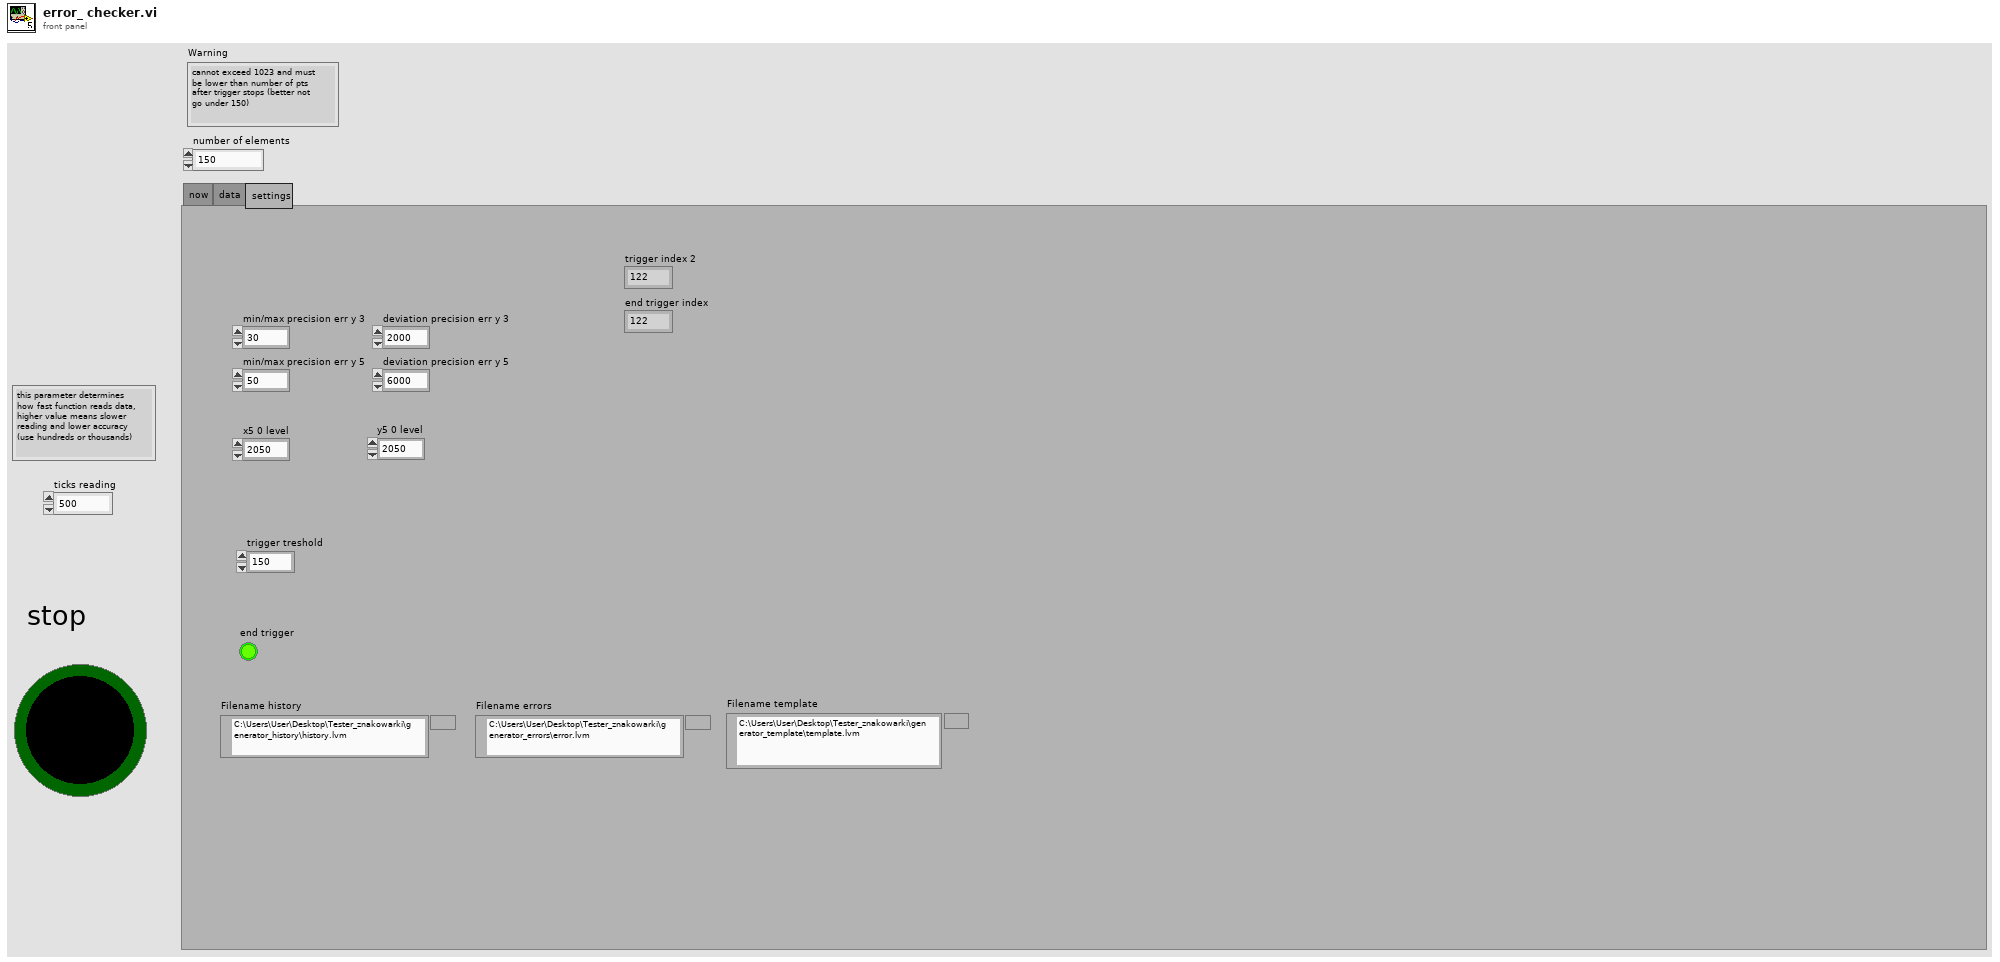
[diagram p1: front panel]
types:
  T1 = cluster{"time":i32[], "gathered err y 5":i16[]}[]
  T2 = cluster{"time":i32[], "template err x 3":i16[]}[]
  T3 = cluster{"time":i32[], "gathered err x 5":i16[]}[]
  T4 = cluster{"num of elem array":i32[], "error y 3 now":i16[]}
  T5 = cluster{"num of elem array":i32[], "error y 5 now":i16[]}
  T6 = cluster{"num of elem array":i32[], "error x 3 now":i16[]}
  T7 = cluster{"num of elem array":i32[], "error x 5 now":i16[]}
  T8 = cluster{"num of elem array":i32[], "error y 5 now":i16[]}[]
  T9 = cluster{"num of elem array":i32[], "error x 5 now":i16[]}[]
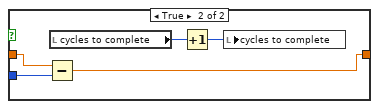
[diagram p3: hidden frame]
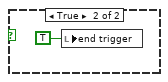
[diagram p5: hidden frame]
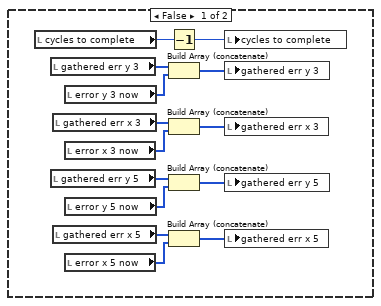
[diagram p6: hidden frame]
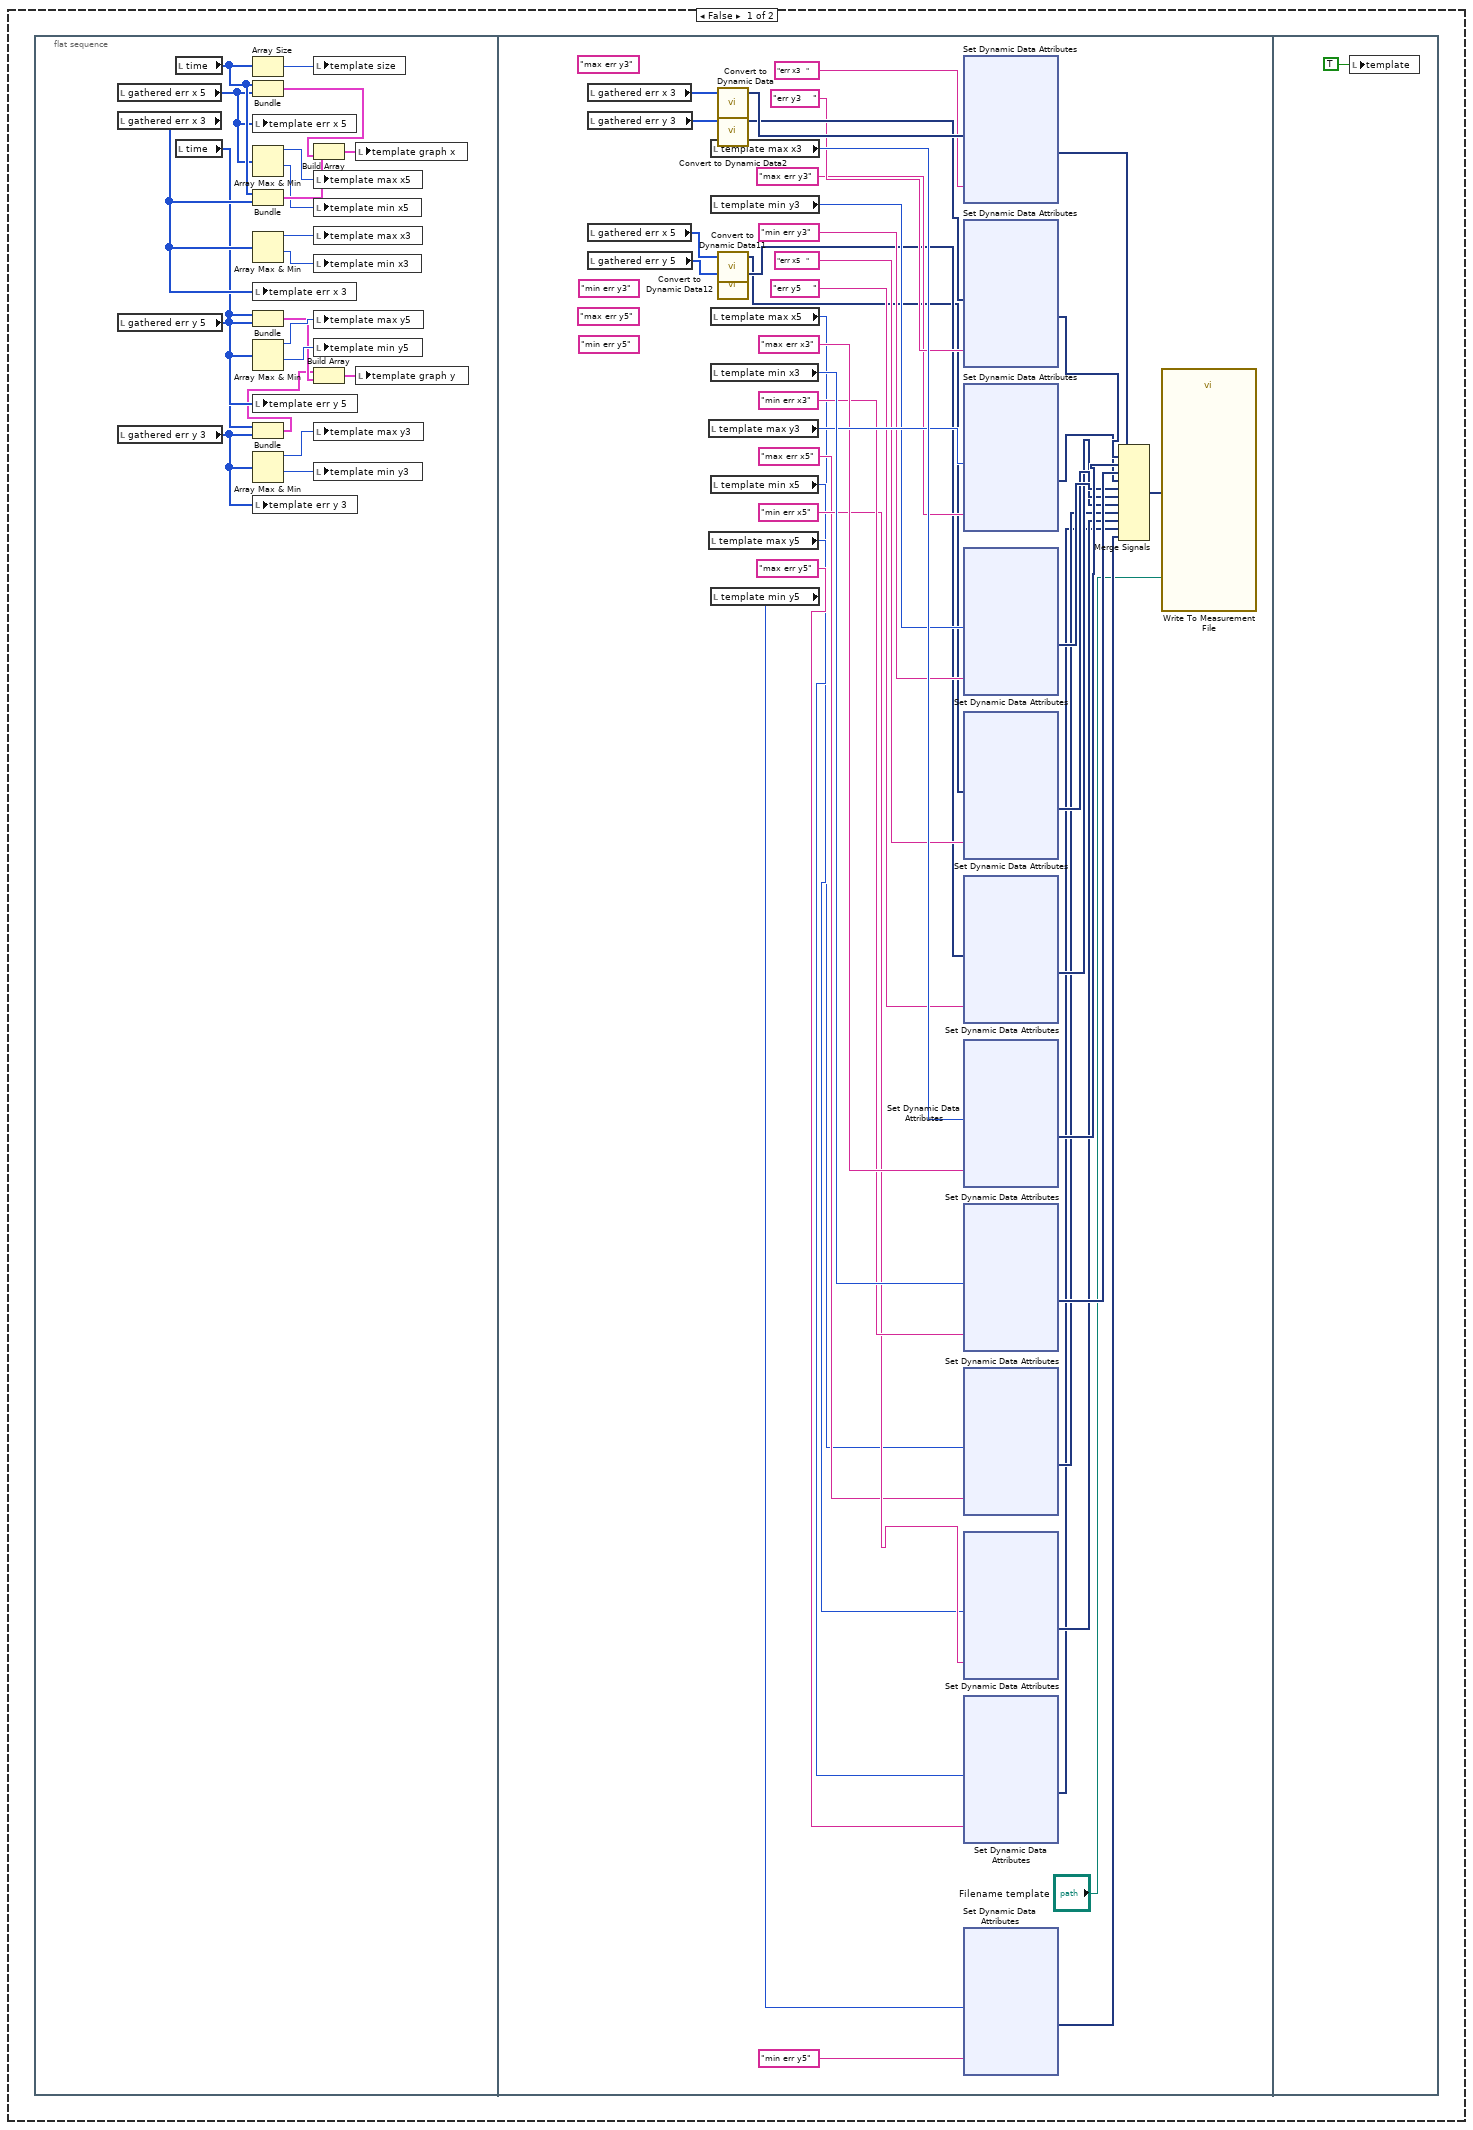
[diagram p7: hidden frame]
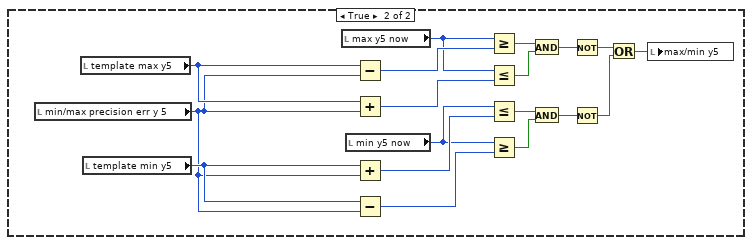
[diagram p8: hidden frame]
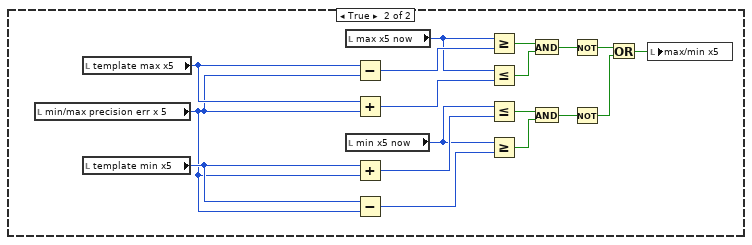
[diagram p9: hidden frame]
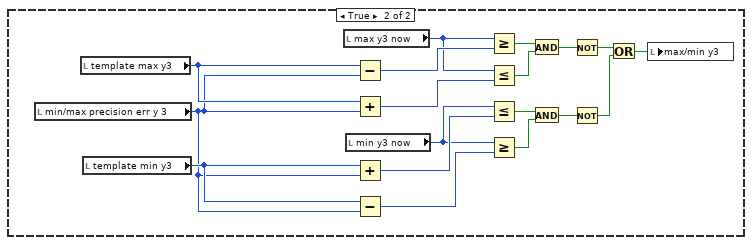
[diagram p10: hidden frame]
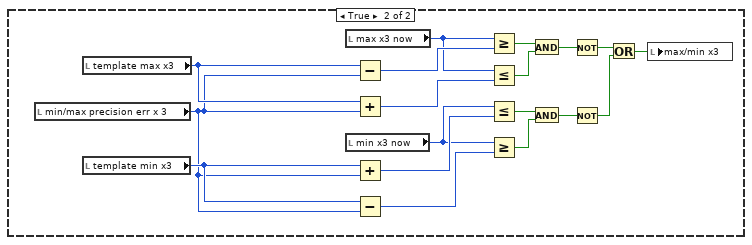
[diagram p11: hidden frame]
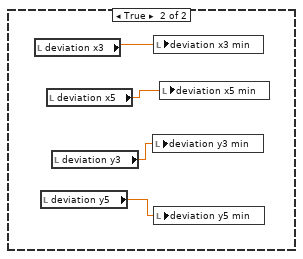
[diagram p12: hidden frame]
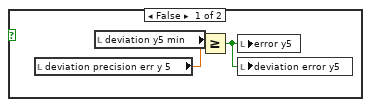
[diagram p13: hidden frame]
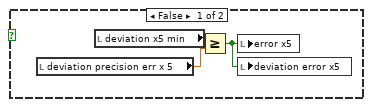
[diagram p14: hidden frame]
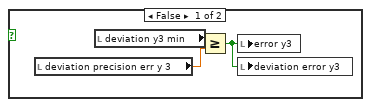
[diagram p15: hidden frame]
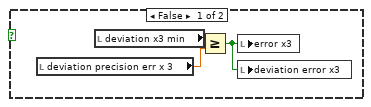
[diagram p16: hidden frame]
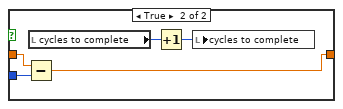
[diagram p19: hidden frame]
diagram:
  n1 = flat-sequence {
    tunnel: [w28] -> w18
    tunnel: [w27] -> w17
    frame #0 {
      w21 = FALSE ("error x now")
      w20 = u16 0 ("Numeric")
      n2 = local write "time"("reset") -> ()
      n3 = local write "stop"(w21) -> ()
      n4 = local write "error y 5 now"("reset") -> ()
      n5 = local write "gathered err x 3"("reset") -> ()
      n6 = local write "error y 3 now"("reset") -> ()
      n7 = local write "gathered err y 3"("reset") -> ()
      n8 = local write "error x 5 now"("reset") -> ()
      n9 = local write "gathered err x 5"("reset") -> ()
      n10 = local write "gathered err y 5"("reset") -> ()
      n11 = local write "num of elem array"("reset") -> ()
      n12 = local write "error x 3 now"("reset") -> ()
      n13 = local write "template err x 3"("reset") -> ()
      n14 = local write "template err y 3"("reset") -> ()
      "trigger" <- w21
      "end trigger" <- w21
      "template" <- w21
      "max/min y3" <- w21
      "max/min x3" <- w21
      "error y3" <- w21
      "error x3" <- w21
      "size now" <- w20
      "template max x3" <- w20
      "template min x3" <- w20
      "template min y3" <- w20
      "max x3 now" <- w20
      "min x3 now" <- w20
      "max y3 now" <- w20
      "min y3 now" <- w20
      "template size" <- w20
      "template max y3" <- w20
      "trigger count" <- w20
      "deviation x3" <- w20
      "deviation y3" <- w20
      "deviation error y3" <- w21
      "deviation error x3" <- w21
      "cycles to complete" <- w20
      "gen size checker" <- 0
      "template max y5" <- w20
      "template min y5" <- w20
      "template min x5" <- w20
      "template max x5" <- w20
      "max y5 now" <- w20
      "max x5 now" <- w20
      "min y5 now" <- w20
      "min x5 now" <- w20
      "max/min x5" <- w21
      "error y5" <- w21
      "error x5" <- w21
      "deviation error x5" <- w21
      "deviation error y5" <- w21
      "max/min y5" <- w21
      "deviation x5" <- w20
      "deviation y5" <- w20
      "deviation x3 min" <- w20
      "deviation x5 min" <- w20
      "deviation y3 min" <- w20
      "deviation y5 min" <- w20
    }
    frame #1 {
      n15 = local read "number of elements"() -> (w25:u32)
      n16 = for {
        N: w25 -> [_]
        tunnel: [w26] -> w24 mode=indexing
        i -> [w26]
      }
      n17 = local write "num of elem array"(w24) -> ()
    }
    frame #2 {
      n18 = xnode "Open FPGA VI Reference"("resource name"=tag "rio://172.22.11.2/RIO0") -> ("FPGA VI Reference Out"=w28:refnum<k20>, "error out"=w27:errorcluster)  [unwired: 1 in]
    }
  }
  n19 = local read "gathered err y 3"() -> (w2:i16[])
  n20 = local read "gathered err y 5"() -> (w1:i16[])
  n21 = local read "template err x 5"() -> (w13:i16[])
  n22 = local read "template err x 3"() -> (w14:i16[])
  n23 = local read "time"() -> (w3:i32[])
  n24 = local read "time"() -> (w12:i32[])
  n25 = Bundle("time"=w3, "gathered err y 3"=w2) -> (w6:cluster{"time":i32[], "gathered err y 3":i16[]})  [unwired: 1 in]
  n26 = Bundle("time"=w3, "gathered err y 5"=w1) -> (w5:cluster{"time":i32[], "gathered err y 5":i16[]})  [unwired: 1 in]
  n27 = Bundle("time"=w12, "template err x 5"=w13) -> (w9:cluster{"time":i32[], "template err x 5":i16[]})  [unwired: 1 in]
  n28 = Bundle("time"=w12, "template err x 3"=w14) -> (w10:cluster{"time":i32[], "template err x 3":i16[]})  [unwired: 1 in]
  n29 = Build Array(w6, w5) -> (w4:T1)
  n30 = Build Array(w9, w10) -> (w11:T2)
  n31 = local write "template graph y"(w4) -> ()
  n32 = local write "template graph x"(w11) -> ()
  n33 = xnode "Invoke Method"("FPGA VI Reference In"=w18, "error in"=w17, "Requested Depth"=u32 1024) -> ("FPGA VI Reference Out"=w8:refnum<k20>, "error out"=w7:errorcluster)  [unwired: 1 out]
  n34 = while {
    tunnel: w8 -> [w40]
    tunnel: w7 -> [w39]
    tunnel: [w38] -> w16
    tunnel: [w37] -> w15
    stop <- "stop" stop-if-true
    n35 = flat-sequence {
      frame #0 {
        n36 = local read "gathered err x 3"() -> (w43:i16[])
        n37 = Array Size(array=w43) -> (size(s)=w42:i32)
        n38 = for {
          N: w42 -> [_]
          tunnel: [w44] -> w41 mode=indexing
          i -> [w44]
        }
        n39 = local write "time"(w41) -> ()
      }
      frame #1 {
        n40 = local read "gathered err y 3"() -> (w48:i16[])
        n41 = local read "gathered err y 5"() -> (w47:i16[])
        n42 = local read "gathered err x 3"() -> (w52:i16[])
        n43 = local read "gathered err x 5"() -> (w53:i16[])
        n44 = local read "time"() -> (w46:i32[])
        n45 = Bundle("time"=w46, "gathered err y 3"=w48) -> (w49:cluster{"time":i32[], "gathered err y 3":i16[]})  [unwired: 1 in]
        n46 = Bundle("time"=w46, "gathered err y 5"=w47) -> (w50:cluster{"time":i32[], "gathered err y 5":i16[]})  [unwired: 1 in]
        n47 = Bundle("time"=w46, "gathered err x 3"=w52) -> (w54:cluster{"time":i32[], "gathered err x 3":i16[]})  [unwired: 1 in]
        n48 = Bundle("time"=w46, "gathered err x 5"=w53) -> (w55:cluster{"time":i32[], "gathered err x 5":i16[]})  [unwired: 1 in]
        n49 = Build Array(w49, w50) -> (w45:T1)
        n50 = Build Array(w54, w55) -> (w51:T3)
        n51 = local write "gathered error y graph"(w45) -> ()
        n52 = local write "gathered error x graph"(w51) -> ()
      }
    }
    n53 = local read "ticks reading"() -> (w32:u32)
    n54 = local read "number of elements"() -> (w31:u32)
    n55 = xnode "Read/Write Control"("FPGA VI Reference In"=w40, "error in"=w39, "count ticks reading"=w32) -> ("FPGA VI Reference Out"=w34:refnum<k20>, "error out"=w33:errorcluster)
    n56 = xnode "Invoke Method"("FPGA VI Reference In"=w34, "error in"=w33, "Number of Elements"=w31, "Timeout (ms)"=-1) -> ("FPGA VI Reference Out"=w38:refnum<k20>, "error out"=w37:errorcluster, "Data"=w35:u64[])  [unwired: 1 out]
    n57 = flat-sequence {
      tunnel: w35 -> [w66]
      frame #0 {
        n58 = Split Number(x=w66) -> (hi(x)=w65:u32[], lo(x)=w64:u32[])
        n59 = Split Number(x=w65) -> (hi(x)=w60:u16[], lo(x)=w58:u16[])
        n60 = Split Number(x=w64) -> (hi(x)=w63:u16[], lo(x)=w62:u16[])
        n61 = To Word Integer(number=w60) -> (16bit integer=→"error x 5 now":i16[])
        n62 = To Word Integer(number=w58) -> (16bit integer=→"error y 5 now":i16[])
        n63 = To Word Integer(number=w63) -> (16bit integer=→"error x 3 now":i16[])
        n64 = To Word Integer(number=w62) -> (16bit integer=→"error y 3 now":i16[])
      }
      frame #1 {
        n65 = local read "num of elem array"() -> (w78:i32[])
        n66 = local read "num of elem array"() -> (w67:i32[])
        n67 = local read "error y 3 now"() -> (w76:i16[])
        n68 = local read "error y 5 now"() -> (w77:i16[])
        n69 = local read "error x 3 now"() -> (w69:i16[])
        n70 = local read "error x 5 now"() -> (w68:i16[])
        n71 = Bundle("num of elem array"=w78, "error y 3 now"=w76) -> (w75:T4)  [unwired: 1 in]
        n72 = Bundle("num of elem array"=w78, "error y 5 now"=w77) -> (w74:T5)  [unwired: 1 in]
        n73 = Bundle("num of elem array"=w67, "error x 3 now"=w69) -> (w70:T6)  [unwired: 1 in]
        n74 = Bundle("num of elem array"=w67, "error x 5 now"=w68) -> (w71:T7)  [unwired: 1 in]
        n75 = Build Array(w75, w74) -> (w73:T8)
        n76 = Build Array(w70, w71) -> (w72:T9)
        n77 = local write "error y graph current elements"(w73) -> ()
        n78 = local write "error x graph current elements"(w72) -> ()
      }
      frame #2 {
        n79 = local read "trigger"() -> (w79:bool)
        n80 = case shown="False" w79 {
          frame False {
            n81 = flat-sequence {
              frame #0 {
                n82 = local read "number of elements"() -> (w80:u32)
                n83 = for {
                  N: w80 -> [_]
                  i -> [w93]
                  stop <- w92 stop-if-true
                  n84 = local read "error y 5 now"() -> (w94:i16[])
                  n85 = local read "error x 5 now"() -> (w95:i16[])
                  n86 = Index Array(array=w95, index=w93) -> (element=w90:i16)
                  n87 = Index Array(array=w94, index=w93) -> (element=w88:i16)
                  n88 = Subtract(x=w90, y="x5 0 level") -> (x-y=w87:i16)
                  n89 = Subtract(x=w88, y="y5 0 level") -> (x-y=w85:i16)
                  n90 = Absolute Value(x=w85) -> (abs(x)=w84:i16)
                  n91 = Greater?(x=w84, y="trigger treshold") -> (0:w81:bool)
                  n92 = Absolute Value(x=w87) -> (abs(x)=w86:i16)
                  n93 = Greater?(x=w86, y="trigger treshold") -> (0:w82:bool)
                  n94 = Or(x=w82, y=w81) -> (x .or. y?=w92:bool)
                  n95 = local write "trigger"(w92) -> ()
                  "trigger index" <- w93
                }
              }
              frame #1 {
                n96 = local read "trigger"() -> (w96:bool)
                n97 = case shown="True" w96 {
                  frame False {
                  }
                  frame True {
                    n98 = flat-sequence {
                      frame #0 {
                        n99 = local read "reset"() -> (w97:i16[])
                        n100 = local read "trigger count"() -> (w99:i16)
                        n101 = local write "gathered err x 3"(w97) -> ()
                        n102 = local write "gathered err y 3"(w97) -> ()
                        n103 = local write "gathered err x 5"(w97) -> ()
                        n104 = local write "gathered err y 5"(w97) -> ()
                        n105 = Increment(x=w99) -> (x+1=w98:i16)
                        n106 = local write "trigger count"(w98) -> ()
                      }
                      frame #1 {
                        n107 = local read "number of elements"() -> (w109:u32)
                        n108 = Divide(x="number of pts after trigger stops", y=w109) -> (x/y=w108:dbl)
                        n109 = Round Toward -Infinity(1:w108) -> (0:w100:dbl)
                        n110 = Multiply(x=w100, y=w109) -> (x*y=w106:dbl)
                        n111 = local write "cycles to complete"(w100) -> ()
                        n112 = local read "trigger index"() -> (w104:i32)
                        "trigger index 2" <- w104
                        n113 = Subtract(x="number of pts after trigger stops", y=w106) -> (x-y=w105:dbl)
                        n114 = Add(x=w105, y=w104) -> (x+y=w102:dbl)
                        n115 = Greater Or Equal?(x=w102, y=w109) -> (x >= y?=w103:bool)
                        n116 = case shown="False" w103 {
                          tunnel: w102 -> [w110 w113]
                          tunnel: [w110 w112] -> w101
                          tunnel: w109 -> [_ w111]
                          frame False {
                          }
                          frame True {
                            n117 = Subtract(x=w113, y=w111) -> (x-y=w112:dbl)
                            n118 = local read "cycles to complete"() -> (w115:i32)
                            n119 = Increment(x=w115) -> (x+1=w114:i32)
                            n120 = local write "cycles to complete"(w114) -> ()
                          }
                        }
                        "end trigger index" <- w101
                      }
                      frame #2 {
                        n121 = local read "cycles to complete"() -> (w128:i32)
                        n122 = local read "number of elements"() -> (w130:u32)
                        n123 = local read "number of elements"() -> (w125:u32)
                        n124 = local read "trigger index"() -> (w129:i32)
                        n125 = local read "trigger index"() -> (w126:i32)
                        n126 = local read "error y 3 now"() -> (w138:i16[])
                        n127 = local read "error y 5 now"() -> (w117:i16[])
                        n128 = local read "error x 3 now"() -> (w139:i16[])
                        n129 = local read "error x 5 now"() -> (w116:i16[])
                        n130 = Decrement(x=w128) -> (x-1=w127:i32)
                        n131 = local read "gathered err y 3"() -> (w136:i16[])
                        n132 = local read "gathered err x 3"() -> (w132:i16[])
                        n133 = local read "gathered err y 5"() -> (w119:i16[])
                        n134 = local read "gathered err x 5"() -> (w123:i16[])
                        n135 = Subtract(x=w130, y=w129) -> (x-y=w137:u32)
                        n136 = Subtract(x=w125, y=w126) -> (x-y=w118:u32)
                        n137 = local write "cycles to complete"(w127) -> ()
                        n138 = Array Subset(array=w138, index=w129, length=w137) -> (w134:i16[])
                        n139 = Array Subset(array=w139, index=w129, length=w137) -> (w133:i16[])
                        n140 = Array Subset(array=w117, index=w126, length=w118) -> (w121:i16[])
                        n141 = Array Subset(array=w116, index=w126, length=w118) -> (w122:i16[])
                        n142 = Build Array (concatenate)(w136, w134) -> (w135:i16[])
                        n143 = Build Array (concatenate)(w132, w133) -> (w131:i16[])
                        n144 = Build Array (concatenate)(w119, w121) -> (w120:i16[])
                        n145 = Build Array (concatenate)(w123, w122) -> (w124:i16[])
                        n146 = local write "gathered err y 3"(w135) -> ()
                        n147 = local write "gathered err x 3"(w131) -> ()
                        n148 = local write "gathered err y 5"(w120) -> ()
                        n149 = local write "gathered err x 5"(w124) -> ()
                      }
                    }
                  }
                }
              }
            }
          }
          frame True {
            n150 = flat-sequence {
              frame #0 {
                n151 = local read "cycles to complete"() -> (w140:i32)
                n152 = Equal?(x=0.0, y=w140) -> (x = y?=w142:bool)
                n153 = case shown="False" w142 {
                  frame False {
                    n154 = local write "end trigger"(FALSE ("end trigger")) -> ()
                  }
                  frame True {
                    n155 = local write "end trigger"(TRUE ("end trigger")) -> ()
                  }
                }
              }
              frame #1 {
                n156 = local read "end trigger"() -> (w145:bool)
                n157 = case shown="True" w145 {
                  frame False {
                    n158 = local read "cycles to complete"() -> (w153:i32)
                    n159 = local read "gathered err y 3"() -> (w155:i16[])
                    n160 = local read "gathered err y 5"() -> (w150:i16[])
                    n161 = local read "gathered err x 3"() -> (w158:i16[])
                    n162 = local read "gathered err x 5"() -> (w147:i16[])
                    n163 = local read "error y 3 now"() -> (w154:i16[])
                    n164 = local read "error x 3 now"() -> (w159:i16[])
                    n165 = local read "error y 5 now"() -> (w151:i16[])
                    n166 = local read "error x 5 now"() -> (w146:i16[])
                    n167 = Decrement(x=w153) -> (x-1=w152:i32)
                    n168 = Build Array (concatenate)(w155, w154) -> (w156:i16[])
                    n169 = Build Array (concatenate)(w158, w159) -> (w157:i16[])
                    n170 = Build Array (concatenate)(w150, w151) -> (w149:i16[])
                    n171 = Build Array (concatenate)(w147, w146) -> (w148:i16[])
                    n172 = local write "cycles to complete"(w152) -> ()
                    n173 = local write "gathered err y 3"(w156) -> ()
                    n174 = local write "gathered err x 3"(w157) -> ()
                    n175 = local write "gathered err y 5"(w149) -> ()
                    n176 = local write "gathered err x 5"(w148) -> ()
                  }
                  frame True {
                    n177 = flat-sequence {
                      frame #0 {
                        w161 = 0 ("index")
                        w178 = 0 ("index")
                        n178 = local read "end trigger index"() -> (w179:i32)
                        n179 = local read "end trigger index"() -> (w160:i32)
                        n180 = local read "error y 3 now"() -> (w177:i16[])
                        n181 = local read "error x 3 now"() -> (w176:i16[])
                        n182 = local read "error y 5 now"() -> (w162:i16[])
                        n183 = local read "error x 5 now"() -> (w163:i16[])
                        n184 = local read "gathered err y 3"() -> (w173:i16[])
                        n185 = local read "gathered err y 5"() -> (w166:i16[])
                        n186 = local read "gathered err x 3"() -> (w172:i16[])
                        n187 = local read "gathered err x 5"() -> (w167:i16[])
                        n188 = Array Subset(array=w177, index=w178, length=w179) -> (w174:i16[])
                        n189 = Array Subset(array=w176, index=w178, length=w179) -> (w175:i16[])
                        n190 = Array Subset(array=w162, index=w161, length=w160) -> (w165:i16[])
                        n191 = Array Subset(array=w163, index=w161, length=w160) -> (w164:i16[])
                        n192 = Build Array (concatenate)(w173, w174) -> (w171:i16[])
                        n193 = Build Array (concatenate)(w172, w175) -> (w170:i16[])
                        n194 = Build Array (concatenate)(w166, w165) -> (w168:i16[])
                        n195 = Build Array (concatenate)(w167, w164) -> (w169:i16[])
                        n196 = local write "gathered err y 3"(w171) -> ()
                        n197 = local write "gathered err x 3"(w170) -> ()
                        n198 = local write "gathered err y 5"(w168) -> ()
                        n199 = local write "gathered err x 5"(w169) -> ()
                      }
                      frame #1 {
                        n200 = local read "gathered err x 3"() -> (w182:i16[])
                        n201 = Array Size(array=w182) -> (size(s)=w181:i32)
                        n202 = for {
                          N: w181 -> [_]
                          tunnel: [w183] -> w180 mode=indexing
                          i -> [w183]
                        }
                        n203 = local write "time"(w180) -> ()
                      }
                      frame #2 {
                        n204 = local write "trigger"(FALSE ("end trigger")) -> ()
                        n205 = local read "gathered err y 3"() -> (w186:i16[])
                        n206 = local read "gathered err y 5"() -> (w185:i16[])
                        n207 = local read "gathered err x 3"() -> (w193:i16[])
                        n208 = local read "gathered err x 5"() -> (w194:i16[])
                        n209 = local read "time"() -> (w184:i32[])
                        n210 = local read "time"() -> (w195:i32[])
                        n211 = Bundle("time"=w184, "gathered err y 3"=w186) -> (w187:cluster{"time":i32[], "gathered err y 3":i16[]})  [unwired: 1 in]
                        n212 = Bundle("time"=w184, "gathered err y 5"=w185) -> (w188:cluster{"time":i32[], "gathered err y 5":i16[]})  [unwired: 1 in]
                        n213 = Bundle("time"=w195, "gathered err x 3"=w193) -> (w192:cluster{"time":i32[], "gathered err x 3":i16[]})  [unwired: 1 in]
                        n214 = Bundle("time"=w195, "gathered err x 5"=w194) -> (w191:cluster{"time":i32[], "gathered err x 5":i16[]})  [unwired: 1 in]
                        n215 = Build Array(w187, w188) -> (w189:T1)
                        n216 = Build Array(w192, w191) -> (w190:T3)
                        n217 = local write "gathered error y graph"(w189) -> ()
                        n218 = local write "gathered error x graph"(w190) -> ()
                      }
                      frame #3 {
                        n219 = local read "template"() -> (w197:bool)
                        n220 = case shown="True" w197 {
                          frame False {
                            n221 = flat-sequence {
                              frame #0 {
                                n222 = local read "gathered err x 5"() -> (w208:i16[])
                                n223 = local read "gathered err x 3"() -> (w209:i16[])
                                n224 = local read "gathered err y 5"() -> (w207:i16[])
                                n225 = local read "gathered err y 3"() -> (w206:i16[])
                                n226 = local read "time"() -> (w215:i32[])
                                n227 = local read "time"() -> (w201:i32[])
                                n228 = Array Size(array=w215) -> (size(s)=w214:i32)
                                n229 = Bundle("time"=w215, "gathered err x 5"=w208) -> (w217:cluster{"time":i32[], "gathered err x 5":i16[]})  [unwired: 1 in]
                                n230 = local write "template err x 5"(w208) -> ()
                                n231 = Array Max & Min(array=w208) -> (max value=w211:i16, min value=w210:i16)  [unwired: 2 out]
                                n232 = Bundle("time"=w215, "gathered err x 3"=w209) -> (w218:cluster{"time":i32[], "gathered err x 3":i16[]})  [unwired: 1 in]
                                n233 = Array Max & Min(array=w209) -> (max value=w213:i16, min value=w212:i16)  [unwired: 2 out]
                                n234 = local write "template err x 3"(w209) -> ()
                                n235 = Bundle("time"=w201, "gathered err y 5"=w207) -> (w199:cluster{"time":i32[], "gathered err y 5":i16[]})  [unwired: 1 in]
                                n236 = Array Max & Min(array=w207) -> (max value=w204:i16, min value=w205:i16)  [unwired: 2 out]
                                n237 = local write "template err y 5"(w207) -> ()
                                n238 = Bundle("time"=w201, "gathered err y 3"=w206) -> (w198:cluster{"time":i32[], "gathered err y 3":i16[]})  [unwired: 1 in]
                                n239 = Array Max & Min(array=w206) -> (max value=w202:i16, min value=w203:i16)  [unwired: 2 out]
                                n240 = local write "template err y 3"(w206) -> ()
                                n241 = local write "template size"(w214) -> ()
                                n242 = Build Array(w218, w217) -> (w216:T3)
                                n243 = local write "template max x5"(w211) -> ()
                                n244 = local write "template min x5"(w210) -> ()
                                n245 = local write "template max x3"(w213) -> ()
                                n246 = local write "template min x3"(w212) -> ()
                                n247 = local write "template max y5"(w204) -> ()
                                n248 = local write "template min y5"(w205) -> ()
                                n249 = Build Array(w198, w199) -> (w200:T1)
                                n250 = local write "template max y3"(w202) -> ()
                                n251 = local write "template min y3"(w203) -> ()
                                n252 = local write "template graph x"(w216) -> ()
                                n253 = local write "template graph y"(w200) -> ()
                              }
                              frame #1 {
                                (unwired) "min err y5" ("Signal Name")
                                (unwired) "max err y5" ("Signal Name")
                                (unwired) "min err y3" ("Signal Name")
                                (unwired) "max err y3" ("Signal Name")
                                n254 = local read "gathered err x 3"() -> (w260:i16[])
                                n255 = local read "gathered err y 3"() -> (w258:i16[])
                                n256 = local read "gathered err x 5"() -> (w227:i16[])
                                n257 = local read "gathered err y 5"() -> (w229:i16[])
                                n258 = local read "template max y3"() -> (w249:i16)
                                n259 = local read "template max y5"() -> (w233:i16)
                                n260 = local read "template max x3"() -> (w254:i16)
                                n261 = local read "template min y3"() -> (w248:i16)
                                n262 = local read "template max x5"() -> (w231:i16)
                                n263 = local read "template min x3"() -> (w252:i16)
                                n264 = local read "template min x5"() -> (w232:i16)
                                n265 = local read "template min y5"() -> (w234:i16)
                                n266 = call "Convert to Dynamic Data"("Array"=w260) -> ("Dynamic Data Type"=w259:dynamicdata)  [unwired: 3 in]
                                n267 = call "Convert to Dynamic Data2"("Array"=w258) -> ("Dynamic Data Type"=w257:dynamicdata)  [unwired: 3 in]
                                n268 = call "Convert to Dynamic Data11"("Array"=w227) -> ("Dynamic Data Type"=w228:dynamicdata)  [unwired: 3 in]
                                n269 = call "Convert to Dynamic Data12"("Array"=w229) -> ("Dynamic Data Type"=w230:dynamicdata)  [unwired: 3 in]
                                n270 = xnode "Set Dynamic Data Attributes"("Signals In"=w259, "Signal Name"="err x3   ") -> ("Signals Out"=w255:dynamicdata)  [unwired: 2 in, 1 out]
                                n271 = xnode "Set Dynamic Data Attributes"("Signals In"=w257, "Signal Name"="err y3    ") -> ("Signals Out"=w256:dynamicdata)  [unwired: 2 in, 1 out]
                                n272 = xnode "Set Dynamic Data Attributes"("Signals In"=w249, "Signal Name"="max err y3") -> ("Signals Out"=w250:dynamicdata)  [unwired: 2 in, 1 out]
                                n273 = xnode "Set Dynamic Data Attributes"("Signals In"=w248, "Signal Name"="min err y3") -> ("Signals Out"=w247:dynamicdata)  [unwired: 2 in, 1 out]
                                n274 = xnode "Set Dynamic Data Attributes"("Signals In"=w228, "Signal Name"="err x5   ") -> ("Signals Out"=w226:dynamicdata)  [unwired: 2 in, 1 out]
                                n275 = xnode "Set Dynamic Data Attributes"("Signals In"=w230, "Signal Name"="err y5    ") -> ("Signals Out"=w225:dynamicdata)  [unwired: 2 in, 1 out]
                                n276 = xnode "Set Dynamic Data Attributes"("Signals In"=w254, "Signal Name"="max err x3") -> ("Signals Out"=w253:dynamicdata)  [unwired: 2 in, 1 out]
                                n277 = xnode "Set Dynamic Data Attributes"("Signals In"=w252, "Signal Name"="min err x3") -> ("Signals Out"=w251:dynamicdata)  [unwired: 2 in, 1 out]
                                n278 = xnode "Set Dynamic Data Attributes"("Signals In"=w231, "Signal Name"="max err x5") -> ("Signals Out"=w224:dynamicdata)  [unwired: 2 in, 1 out]
                                n279 = xnode "Set Dynamic Data Attributes"("Signals In"=w232, "Signal Name"="min err x5") -> ("Signals Out"=w223:dynamicdata)  [unwired: 2 in, 1 out]
                                n280 = xnode "Set Dynamic Data Attributes"("Signals In"=w233, "Signal Name"="max err y5") -> ("Signals Out"=w222:dynamicdata)  [unwired: 2 in, 1 out]
                                n281 = xnode "Set Dynamic Data Attributes"("Signals In"=w234, "Signal Name"="min err y5") -> ("Signals Out"=w221:dynamicdata)  [unwired: 2 in, 1 out]
                                n282 = Merge Signals(w255, w256, w253, w251, w250, w247, w226, w225, w224, w223, w222, w221) -> (w220:dynamicdata)
                                n283 = call "Write To Measurement File"("Signals"=w220, "Filename"="Filename template") -> ()  [unwired: 15 in, 3 out]
                              }
                              frame #2 {
                                n284 = local write "template"(TRUE ("template")) -> ()
                              }
                            }
                          }
                          frame True {
                            n285 = flat-sequence {
                              frame #0 {
                                n286 = local read "time"() -> (w436:i32[])
                                n287 = local read "gathered err y 3"() -> (w442:i16[])
                                n288 = local read "gathered err x 3"() -> (w443:i16[])
                                n289 = local read "gathered err y 5"() -> (w431:i16[])
                                n290 = local read "gathered err x 5"() -> (w430:i16[])
                                n291 = Array Size(array=w436) -> (size(s)=w437:i32)
                                n292 = local write "size now"(w437) -> ()
                                n293 = Array Max & Min(array=w442) -> (max value=w439:i16, min value=w438:i16)  [unwired: 2 out]
                                n294 = Array Max & Min(array=w443) -> (max value=w441:i16, min value=w440:i16)  [unwired: 2 out]
                                n295 = Array Max & Min(array=w431) -> (max value=w434:i16, min value=w435:i16)  [unwired: 2 out]
                                n296 = Array Max & Min(array=w430) -> (max value=w432:i16, min value=w433:i16)  [unwired: 2 out]
                                n297 = local write "max y3 now"(w439) -> ()
                                n298 = local write "min y3 now"(w438) -> ()
                                n299 = local write "max x3 now"(w441) -> ()
                                n300 = local write "min x3 now"(w440) -> ()
                                n301 = local write "max y5 now"(w434) -> ()
                                n302 = local write "min y5 now"(w435) -> ()
                                n303 = local write "max x5 now"(w432) -> ()
                                n304 = local write "min x5 now"(w433) -> ()
                              }
                              frame #1 {
                                n305 = local read "error y3"() -> (w447:bool)
                                n306 = local read "error y5"() -> (w444:bool)
                                n307 = local read "error x3"() -> (w446:bool)
                                n308 = local read "error x5"() -> (w445:bool)
                                n309 = case shown="False" w447 {
                                frame False {
                                n310 = local read "min/max precision err y 3"() -> (w521:i16)
                                n311 = local read "template max y3"() -> (w525:i16)
                                n312 = local read "template min y3"() -> (w523:i16)
                                n313 = local read "max y3 now"() -> (w524:i16)
                                n314 = local read "min y3 now"() -> (w522:i16)
                                n315 = Subtract(x=w525, y=w521) -> (x-y=w530:i16)
                                n316 = Add(x=w525, y=w521) -> (x+y=w531:i16)
                                n317 = Add(x=w523, y=w521) -> (x+y=w529:i16)
                                n318 = Subtract(x=w523, y=w521) -> (x-y=w528:i16)
                                n319 = Greater Or Equal?(x=w524, y=w530) -> (x >= y?=w537:bool)
                                n320 = Less Or Equal?(x=w524, y=w531) -> (x <= y?=w536:bool)
                                n321 = Less Or Equal?(x=w522, y=w529) -> (x <= y?=w534:bool)
                                n322 = Greater Or Equal?(x=w522, y=w528) -> (x >= y?=w533:bool)
                                n323 = And(x=w537, y=w536) -> (x .and. y?=w535:bool)
                                n324 = And(x=w534, y=w533) -> (x .and. y?=w532:bool)
                                n325 = Not(x=w535) -> (.not. x?=w527:bool)
                                n326 = Not(x=w532) -> (.not. x?=w526:bool)
                                n327 = Or(x=w527, y=w526) -> (x .or. y?=w520:bool)
                                n328 = local write "error y3"(w520) -> ()
                                n329 = local write "max/min y3"(w520) -> ()
                                }
                                frame True {
                                n330 = local read "min/max precision err y 3"() -> (w541:i16)
                                n331 = local read "template max y3"() -> (w543:i16)
                                n332 = local read "template min y3"() -> (w542:i16)
                                n333 = local read "max y3 now"() -> (w545:i16)
                                n334 = local read "min y3 now"() -> (w544:i16)
                                n335 = Subtract(x=w543, y=w541) -> (x-y=w548:i16)
                                n336 = Add(x=w543, y=w541) -> (x+y=w549:i16)
                                n337 = Add(x=w542, y=w541) -> (x+y=w547:i16)
                                n338 = Subtract(x=w542, y=w541) -> (x-y=w546:i16)
                                n339 = Greater Or Equal?(x=w545, y=w548) -> (x >= y?=w555:bool)
                                n340 = Less Or Equal?(x=w545, y=w549) -> (x <= y?=w554:bool)
                                n341 = Less Or Equal?(x=w544, y=w547) -> (x <= y?=w552:bool)
                                n342 = Greater Or Equal?(x=w544, y=w546) -> (x >= y?=w551:bool)
                                n343 = And(x=w555, y=w554) -> (x .and. y?=w553:bool)
                                n344 = And(x=w552, y=w551) -> (x .and. y?=w550:bool)
                                n345 = Not(x=w553) -> (.not. x?=w540:bool)
                                n346 = Not(x=w550) -> (.not. x?=w539:bool)
                                n347 = Or(x=w540, y=w539) -> (x .or. y?=w538:bool)
                                n348 = local write "max/min y3"(w538) -> ()
                                }
                                }
                                n349 = case shown="False" w446 {
                                frame False {
                                n350 = local read "min/max precision err x 3"() -> (w559:i16)
                                n351 = local read "template max x3"() -> (w561:i16)
                                n352 = local read "template min x3"() -> (w560:i16)
                                n353 = local read "max x3 now"() -> (w562:i16)
                                n354 = local read "min x3 now"() -> (w563:i16)
                                n355 = Subtract(x=w561, y=w559) -> (x-y=w566:i16)
                                n356 = Add(x=w561, y=w559) -> (x+y=w567:i16)
                                n357 = Add(x=w560, y=w559) -> (x+y=w565:i16)
                                n358 = Subtract(x=w560, y=w559) -> (x-y=w564:i16)
                                n359 = Greater Or Equal?(x=w562, y=w566) -> (x >= y?=w573:bool)
                                n360 = Less Or Equal?(x=w562, y=w567) -> (x <= y?=w572:bool)
                                n361 = Less Or Equal?(x=w563, y=w565) -> (x <= y?=w570:bool)
                                n362 = Greater Or Equal?(x=w563, y=w564) -> (x >= y?=w569:bool)
                                n363 = And(x=w573, y=w572) -> (x .and. y?=w571:bool)
                                n364 = And(x=w570, y=w569) -> (x .and. y?=w568:bool)
                                n365 = Not(x=w571) -> (.not. x?=w557:bool)
                                n366 = Not(x=w568) -> (.not. x?=w558:bool)
                                n367 = Or(x=w557, y=w558) -> (x .or. y?=w556:bool)
                                n368 = local write "error x3"(w556) -> ()
                                n369 = local write "max/min x3"(w556) -> ()
                                }
                                frame True {
                                n370 = local read "min/max precision err x 3"() -> (w574:i16)
                                n371 = local read "template max x3"() -> (w578:i16)
                                n372 = local read "template min x3"() -> (w576:i16)
                                n373 = local read "max x3 now"() -> (w577:i16)
                                n374 = local read "min x3 now"() -> (w575:i16)
                                n375 = Subtract(x=w578, y=w574) -> (x-y=w584:i16)
                                n376 = Add(x=w578, y=w574) -> (x+y=w585:i16)
                                n377 = Add(x=w576, y=w574) -> (x+y=w583:i16)
                                n378 = Subtract(x=w576, y=w574) -> (x-y=w582:i16)
                                n379 = Greater Or Equal?(x=w577, y=w584) -> (x >= y?=w591:bool)
                                n380 = Less Or Equal?(x=w577, y=w585) -> (x <= y?=w590:bool)
                                n381 = Less Or Equal?(x=w575, y=w583) -> (x <= y?=w588:bool)
                                n382 = Greater Or Equal?(x=w575, y=w582) -> (x >= y?=w587:bool)
                                n383 = And(x=w591, y=w590) -> (x .and. y?=w589:bool)
                                n384 = And(x=w588, y=w587) -> (x .and. y?=w586:bool)
                                n385 = Not(x=w589) -> (.not. x?=w580:bool)
                                n386 = Not(x=w586) -> (.not. x?=w581:bool)
                                n387 = Or(x=w580, y=w581) -> (x .or. y?=w579:bool)
                                n388 = local write "max/min x3"(w579) -> ()
                                }
                                }
                                n389 = case shown="False" w444 {
                                frame False {
                                n390 = local read "min/max precision err y 5"() -> (w449:i16)
                                n391 = local read "template max y5"() -> (w453:i16)
                                n392 = local read "template min y5"() -> (w451:i16)
                                n393 = local read "max y5 now"() -> (w452:i16)
                                n394 = local read "min y5 now"() -> (w450:i16)
                                n395 = Subtract(x=w453, y=w449) -> (x-y=w458:i16)
                                n396 = Add(x=w453, y=w449) -> (x+y=w459:i16)
                                n397 = Add(x=w451, y=w449) -> (x+y=w457:i16)
                                n398 = Subtract(x=w451, y=w449) -> (x-y=w456:i16)
                                n399 = Greater Or Equal?(x=w452, y=w458) -> (x >= y?=w465:bool)
                                n400 = Less Or Equal?(x=w452, y=w459) -> (x <= y?=w464:bool)
                                n401 = Less Or Equal?(x=w450, y=w457) -> (x <= y?=w462:bool)
                                n402 = Greater Or Equal?(x=w450, y=w456) -> (x >= y?=w461:bool)
                                n403 = And(x=w465, y=w464) -> (x .and. y?=w463:bool)
                                n404 = And(x=w462, y=w461) -> (x .and. y?=w460:bool)
                                n405 = Not(x=w463) -> (.not. x?=w455:bool)
                                n406 = Not(x=w460) -> (.not. x?=w454:bool)
                                n407 = Or(x=w455, y=w454) -> (x .or. y?=w448:bool)
                                n408 = local write "error y5"(w448) -> ()
                                n409 = local write "max/min y5"(w448) -> ()
                                }
                                frame True {
                                n410 = local read "min/max precision err y 5"() -> (w469:i16)
                                n411 = local read "template max y5"() -> (w471:i16)
                                n412 = local read "template min y5"() -> (w470:i16)
                                n413 = local read "max y5 now"() -> (w473:i16)
                                n414 = local read "min y5 now"() -> (w472:i16)
                                n415 = Subtract(x=w471, y=w469) -> (x-y=w476:i16)
                                n416 = Add(x=w471, y=w469) -> (x+y=w477:i16)
                                n417 = Add(x=w470, y=w469) -> (x+y=w475:i16)
                                n418 = Subtract(x=w470, y=w469) -> (x-y=w474:i16)
                                n419 = Greater Or Equal?(x=w473, y=w476) -> (x >= y?=w483:bool)
                                n420 = Less Or Equal?(x=w473, y=w477) -> (x <= y?=w482:bool)
                                n421 = Less Or Equal?(x=w472, y=w475) -> (x <= y?=w480:bool)
                                n422 = Greater Or Equal?(x=w472, y=w474) -> (x >= y?=w479:bool)
                                n423 = And(x=w483, y=w482) -> (x .and. y?=w481:bool)
                                n424 = And(x=w480, y=w479) -> (x .and. y?=w478:bool)
                                n425 = Not(x=w481) -> (.not. x?=w468:bool)
                                n426 = Not(x=w478) -> (.not. x?=w467:bool)
                                n427 = Or(x=w468, y=w467) -> (x .or. y?=w466:bool)
                                n428 = local write "max/min y5"(w466) -> ()
                                }
                                }
                                n429 = case shown="False" w445 {
                                frame False {
                                n430 = local read "min/max precision err x 5"() -> (w487:i16)
                                n431 = local read "template max x5"() -> (w489:i16)
                                n432 = local read "template min x5"() -> (w488:i16)
                                n433 = local read "max x5 now"() -> (w490:i16)
                                n434 = local read "min x5 now"() -> (w491:i16)
                                n435 = Subtract(x=w489, y=w487) -> (x-y=w494:i16)
                                n436 = Add(x=w489, y=w487) -> (x+y=w495:i16)
                                n437 = Add(x=w488, y=w487) -> (x+y=w493:i16)
                                n438 = Subtract(x=w488, y=w487) -> (x-y=w492:i16)
                                n439 = Greater Or Equal?(x=w490, y=w494) -> (x >= y?=w501:bool)
                                n440 = Less Or Equal?(x=w490, y=w495) -> (x <= y?=w500:bool)
                                n441 = Less Or Equal?(x=w491, y=w493) -> (x <= y?=w498:bool)
                                n442 = Greater Or Equal?(x=w491, y=w492) -> (x >= y?=w497:bool)
                                n443 = And(x=w501, y=w500) -> (x .and. y?=w499:bool)
                                n444 = And(x=w498, y=w497) -> (x .and. y?=w496:bool)
                                n445 = Not(x=w499) -> (.not. x?=w485:bool)
                                n446 = Not(x=w496) -> (.not. x?=w486:bool)
                                n447 = Or(x=w485, y=w486) -> (x .or. y?=w484:bool)
                                n448 = local write "error x5"(w484) -> ()
                                n449 = local write "max/min x5"(w484) -> ()
                                }
                                frame True {
                                n450 = local read "min/max precision err x 5"() -> (w502:i16)
                                n451 = local read "template max x5"() -> (w506:i16)
                                n452 = local read "template min x5"() -> (w504:i16)
                                n453 = local read "max x5 now"() -> (w505:i16)
                                n454 = local read "min x5 now"() -> (w503:i16)
                                n455 = Subtract(x=w506, y=w502) -> (x-y=w512:i16)
                                n456 = Add(x=w506, y=w502) -> (x+y=w513:i16)
                                n457 = Add(x=w504, y=w502) -> (x+y=w511:i16)
                                n458 = Subtract(x=w504, y=w502) -> (x-y=w510:i16)
                                n459 = Greater Or Equal?(x=w505, y=w512) -> (x >= y?=w519:bool)
                                n460 = Less Or Equal?(x=w505, y=w513) -> (x <= y?=w518:bool)
                                n461 = Less Or Equal?(x=w503, y=w511) -> (x <= y?=w516:bool)
                                n462 = Greater Or Equal?(x=w503, y=w510) -> (x >= y?=w515:bool)
                                n463 = And(x=w519, y=w518) -> (x .and. y?=w517:bool)
                                n464 = And(x=w516, y=w515) -> (x .and. y?=w514:bool)
                                n465 = Not(x=w517) -> (.not. x?=w508:bool)
                                n466 = Not(x=w514) -> (.not. x?=w509:bool)
                                n467 = Or(x=w508, y=w509) -> (x .or. y?=w507:bool)
                                n468 = local write "max/min x5"(w507) -> ()
                                }
                                }
                              }
                              frame #2 {
                                n469 = local write "deviation x3"(0.0 ("deviation x")) -> ()
                                n470 = local write "deviation y3"(0.0 ("deviation y")) -> ()
                                n471 = local write "deviation x5"(0.0 ("deviation x")) -> ()
                                n472 = local write "deviation y5"(0.0 ("deviation y")) -> ()
                              }
                              frame #3 {
                                n473 = for {
                                N: 30 -> [_]
                                i -> [w597]
                                n474 = local read "gathered err x 3"() -> (w613:i16[])
                                n475 = local read "template err x 3"() -> (w623:i16[])
                                n476 = local read "gathered err y 3"() -> (w609:i16[])
                                n477 = local read "template err y 3"() -> (w620:i16[])
                                n478 = local read "gathered err x 5"() -> (w605:i16[])
                                n479 = local read "template err x 5"() -> (w616:i16[])
                                n480 = local read "gathered err y 5"() -> (w601:i16[])
                                n481 = local read "template err y 5"() -> (w619:i16[])
                                n482 = Array Size(array=w613) -> (size(s)=w612:i32)
                                n483 = Subtract(x=w612, y=w597) -> (x-y=w611:i32)
                                n484 = Array Size(array=w623) -> (size(s)=w625:i32)
                                n485 = Array Size(array=w609) -> (size(s)=w608:i32)
                                n486 = Subtract(x=w608, y=w597) -> (x-y=w607:i32)
                                n487 = Array Size(array=w620) -> (size(s)=w621:i32)
                                n488 = Array Size(array=w605) -> (size(s)=w604:i32)
                                n489 = Subtract(x=w604, y=w597) -> (x-y=w603:i32)
                                n490 = Array Subset(array=w605, index=w597, length=w603) -> (w602:i16[])
                                n491 = Array Size(array=w616) -> (size(s)=w614:i32)
                                n492 = Array Size(array=w601) -> (size(s)=w600:i32)
                                n493 = Subtract(x=w600, y=w597) -> (x-y=w599:i32)
                                n494 = Array Subset(array=w601, index=w597, length=w599) -> (w598:i16[])
                                n495 = Array Size(array=w619) -> (size(s)=w618:i32)
                                n496 = Array Subset(array=w609, index=w597, length=w607) -> (w606:i16[])
                                n497 = Array Subset(array=w613, index=w597, length=w611) -> (w610:i16[])
                                n498 = Max & Min(x=w611, y=w625) -> (min(x,y)=w624:i32)  [unwired: 1 out]
                                n499 = Max & Min(x=w607, y=w621) -> (min(x,y)=w622:i32)  [unwired: 1 out]
                                n500 = Max & Min(x=w603, y=w614) -> (min(x,y)=w615:i32)  [unwired: 1 out]
                                n501 = Max & Min(x=w599, y=w618) -> (min(x,y)=w617:i32)  [unwired: 1 out]
                                n502 = flat-sequence {
                                tunnel: w624 -> [w637]
                                tunnel: w623 -> [w636]
                                tunnel: w622 -> [w635]
                                tunnel: w620 -> [w634]
                                tunnel: w606 -> [w633]
                                tunnel: w598 -> [w632]
                                tunnel: w619 -> [w631]
                                tunnel: w617 -> [w630]
                                tunnel: w616 -> [w629]
                                tunnel: w615 -> [w628]
                                tunnel: w602 -> [w627]
                                tunnel: w610 -> [w626]
                                tunnel: w597 -> [w687]
                                frame #0 {
                                n503 = for {
                                N: w637 -> [w679]
                                tunnel: w636 -> [w685]
                                tunnel: w626 -> [w684]
                                i -> [w683]
                                n504 = Index Array(array=w685, index=w683) -> (element=w681:i16)
                                n505 = Index Array(array=w684, index=w683) -> (element=w682:i16)
                                n506 = Subtract(x=w682, y=w681) -> (x-y=w675:i16)
                                n507 = To Long Integer(number=w675) -> (32bit integer=w674:i32)
                                n508 = Square(x=w674) -> (x^2=w678:i32)
                                n509 = local read "deviation x3"() -> (w676:dbl)
                                n510 = Divide(x=w678, y=w679) -> (x/y=w677:dbl)
                                n511 = Add(x=w677, y=w676) -> (x+y=w680:dbl)
                                n512 = local write "deviation x3"(w680) -> ()
                                }
                                n513 = for {
                                N: w635 -> [w671]
                                tunnel: w634 -> [w670]
                                tunnel: w633 -> [w669]
                                i -> [w666]
                                n514 = Index Array(array=w669, index=w666) -> (element=w668:i16)
                                n515 = Index Array(array=w670, index=w666) -> (element=w667:i16)
                                n516 = Subtract(x=w668, y=w667) -> (x-y=w663:i16)
                                n517 = To Long Integer(number=w663) -> (32bit integer=w662:i32)
                                n518 = Square(x=w662) -> (x^2=w673:i32)
                                n519 = local read "deviation y3"() -> (w665:dbl)
                                n520 = Divide(x=w673, y=w671) -> (x/y=w672:dbl)
                                n521 = Add(x=w672, y=w665) -> (x+y=w664:dbl)
                                n522 = local write "deviation y3"(w664) -> ()
                                }
                                n523 = for {
                                N: w628 -> [w655]
                                tunnel: w629 -> [w661]
                                tunnel: w627 -> [w660]
                                i -> [w659]
                                n524 = Index Array(array=w660, index=w659) -> (element=w658:i16)
                                n525 = Index Array(array=w661, index=w659) -> (element=w657:i16)
                                n526 = Subtract(x=w658, y=w657) -> (x-y=w651:i16)
                                n527 = To Long Integer(number=w651) -> (32bit integer=w650:i32)
                                n528 = Square(x=w650) -> (x^2=w654:i32)
                                n529 = local read "deviation x5"() -> (w652:dbl)
                                n530 = Divide(x=w654, y=w655) -> (x/y=w653:dbl)
                                n531 = Add(x=w653, y=w652) -> (x+y=w656:dbl)
                                n532 = local write "deviation x5"(w656) -> ()
                                }
                                n533 = for {
                                N: w630 -> [w647]
                                tunnel: w631 -> [w646]
                                tunnel: w632 -> [w645]
                                i -> [w642]
                                n534 = Index Array(array=w645, index=w642) -> (element=w644:i16)
                                n535 = Index Array(array=w646, index=w642) -> (element=w643:i16)
                                n536 = Subtract(x=w644, y=w643) -> (x-y=w639:i16)
                                n537 = To Long Integer(number=w639) -> (32bit integer=w638:i32)
                                n538 = Square(x=w638) -> (x^2=w649:i32)
                                n539 = local read "deviation y5"() -> (w641:dbl)
                                n540 = Divide(x=w649, y=w647) -> (x/y=w648:dbl)
                                n541 = Add(x=w648, y=w641) -> (x+y=w640:dbl)
                                n542 = local write "deviation y5"(w640) -> ()
                                }
                                }
                                frame #1 {
                                n543 = Equal To 0?(x=w687) -> (x = 0?=w686:bool)
                                n544 = case shown="False" w686 {
                                frame False {
                                n545 = local read "deviation y3 min"() -> (w692:dbl)
                                n546 = local read "deviation y5 min"() -> (w689:dbl)
                                n547 = local read "deviation x5 min"() -> (w695:dbl)
                                n548 = local read "deviation x3 min"() -> (w698:dbl)
                                n549 = local read "deviation y5"() -> (w690:dbl)
                                n550 = local read "deviation y3"() -> (w693:dbl)
                                n551 = local read "deviation x5"() -> (w696:dbl)
                                n552 = local read "deviation x3"() -> (w699:dbl)
                                n553 = Max & Min(x=w693, y=w692) -> (min(x,y)=w691:dbl)  [unwired: 1 out]
                                n554 = Max & Min(x=w690, y=w689) -> (min(x,y)=w688:dbl)  [unwired: 1 out]
                                n555 = Max & Min(x=w699, y=w698) -> (min(x,y)=w697:dbl)  [unwired: 1 out]
                                n556 = Max & Min(x=w696, y=w695) -> (min(x,y)=w694:dbl)  [unwired: 1 out]
                                n557 = local write "deviation y3 min"(w691) -> ()
                                n558 = local write "deviation y5 min"(w688) -> ()
                                n559 = local write "deviation x3 min"(w697) -> ()
                                n560 = local write "deviation x5 min"(w694) -> ()
                                }
                                frame True {
                                n561 = local read "deviation x3"() -> (w700:dbl)
                                n562 = local read "deviation y5"() -> (w703:dbl)
                                n563 = local read "deviation x5"() -> (w701:dbl)
                                n564 = local read "deviation y3"() -> (w702:dbl)
                                n565 = local write "deviation y3 min"(w702) -> ()
                                n566 = local write "deviation x3 min"(w700) -> ()
                                n567 = local write "deviation y5 min"(w703) -> ()
                                n568 = local write "deviation x5 min"(w701) -> ()
                                }
                                }
                                }
                                }
                                }
                              }
                              frame #4 {
                                n569 = for {
                                N: 30 -> [_]
                                i -> [w705]
                                n570 = local read "template err x 3"() -> (w721:i16[])
                                n571 = local read "gathered err x 3"() -> (w731:i16[])
                                n572 = local read "template err y 3"() -> (w717:i16[])
                                n573 = local read "gathered err y 3"() -> (w728:i16[])
                                n574 = local read "template err x 5"() -> (w713:i16[])
                                n575 = local read "gathered err x 5"() -> (w724:i16[])
                                n576 = local read "template err y 5"() -> (w709:i16[])
                                n577 = local read "gathered err y 5"() -> (w727:i16[])
                                n578 = Array Size(array=w721) -> (size(s)=w720:i32)
                                n579 = Subtract(x=w720, y=w705) -> (x-y=w719:i32)
                                n580 = Array Size(array=w731) -> (size(s)=w733:i32)
                                n581 = Array Size(array=w717) -> (size(s)=w716:i32)
                                n582 = Subtract(x=w716, y=w705) -> (x-y=w715:i32)
                                n583 = Array Size(array=w728) -> (size(s)=w729:i32)
                                n584 = Array Size(array=w713) -> (size(s)=w712:i32)
                                n585 = Subtract(x=w712, y=w705) -> (x-y=w711:i32)
                                n586 = Array Subset(array=w713, index=w705, length=w711) -> (w710:i16[])
                                n587 = Array Size(array=w724) -> (size(s)=w722:i32)
                                n588 = Array Size(array=w709) -> (size(s)=w708:i32)
                                n589 = Subtract(x=w708, y=w705) -> (x-y=w707:i32)
                                n590 = Array Subset(array=w709, index=w705, length=w707) -> (w706:i16[])
                                n591 = Array Size(array=w727) -> (size(s)=w726:i32)
                                n592 = Array Subset(array=w717, index=w705, length=w715) -> (w714:i16[])
                                n593 = Array Subset(array=w721, index=w705, length=w719) -> (w718:i16[])
                                n594 = Max & Min(x=w719, y=w733) -> (min(x,y)=w732:i32)  [unwired: 1 out]
                                n595 = Max & Min(x=w715, y=w729) -> (min(x,y)=w730:i32)  [unwired: 1 out]
                                n596 = Max & Min(x=w711, y=w722) -> (min(x,y)=w723:i32)  [unwired: 1 out]
                                n597 = Max & Min(x=w707, y=w726) -> (min(x,y)=w725:i32)  [unwired: 1 out]
                                n598 = flat-sequence {
                                tunnel: w732 -> [w745]
                                tunnel: w731 -> [w744]
                                tunnel: w730 -> [w743]
                                tunnel: w728 -> [w742]
                                tunnel: w714 -> [w741]
                                tunnel: w706 -> [w740]
                                tunnel: w727 -> [w739]
                                tunnel: w725 -> [w738]
                                tunnel: w724 -> [w737]
                                tunnel: w723 -> [w736]
                                tunnel: w710 -> [w735]
                                tunnel: w718 -> [w734]
                                frame #0 {
                                n599 = for {
                                N: w745 -> [w787]
                                tunnel: w744 -> [w793]
                                tunnel: w734 -> [w792]
                                i -> [w791]
                                n600 = Index Array(array=w793, index=w791) -> (element=w789:i16)
                                n601 = Index Array(array=w792, index=w791) -> (element=w790:i16)
                                n602 = Subtract(x=w790, y=w789) -> (x-y=w783:i16)
                                n603 = To Long Integer(number=w783) -> (32bit integer=w782:i32)
                                n604 = Square(x=w782) -> (x^2=w786:i32)
                                n605 = local read "deviation x3"() -> (w784:dbl)
                                n606 = Divide(x=w786, y=w787) -> (x/y=w785:dbl)
                                n607 = Add(x=w785, y=w784) -> (x+y=w788:dbl)
                                n608 = local write "deviation x3"(w788) -> ()
                                }
                                n609 = for {
                                N: w743 -> [w779]
                                tunnel: w742 -> [w778]
                                tunnel: w741 -> [w777]
                                i -> [w774]
                                n610 = Index Array(array=w777, index=w774) -> (element=w776:i16)
                                n611 = Index Array(array=w778, index=w774) -> (element=w775:i16)
                                n612 = Subtract(x=w776, y=w775) -> (x-y=w771:i16)
                                n613 = To Long Integer(number=w771) -> (32bit integer=w770:i32)
                                n614 = Square(x=w770) -> (x^2=w781:i32)
                                n615 = local read "deviation y3"() -> (w773:dbl)
                                n616 = Divide(x=w781, y=w779) -> (x/y=w780:dbl)
                                n617 = Add(x=w780, y=w773) -> (x+y=w772:dbl)
                                n618 = local write "deviation y3"(w772) -> ()
                                }
                                n619 = for {
                                N: w736 -> [w763]
                                tunnel: w737 -> [w769]
                                tunnel: w735 -> [w768]
                                i -> [w767]
                                n620 = Index Array(array=w768, index=w767) -> (element=w766:i16)
                                n621 = Index Array(array=w769, index=w767) -> (element=w765:i16)
                                n622 = Subtract(x=w766, y=w765) -> (x-y=w759:i16)
                                n623 = To Long Integer(number=w759) -> (32bit integer=w758:i32)
                                n624 = Square(x=w758) -> (x^2=w762:i32)
                                n625 = local read "deviation x5"() -> (w760:dbl)
                                n626 = Divide(x=w762, y=w763) -> (x/y=w761:dbl)
                                n627 = Add(x=w761, y=w760) -> (x+y=w764:dbl)
                                n628 = local write "deviation x5"(w764) -> ()
                                }
                                n629 = for {
                                N: w738 -> [w755]
                                tunnel: w739 -> [w754]
                                tunnel: w740 -> [w753]
                                i -> [w750]
                                n630 = Index Array(array=w753, index=w750) -> (element=w752:i16)
                                n631 = Index Array(array=w754, index=w750) -> (element=w751:i16)
                                n632 = Subtract(x=w752, y=w751) -> (x-y=w747:i16)
                                n633 = To Long Integer(number=w747) -> (32bit integer=w746:i32)
                                n634 = Square(x=w746) -> (x^2=w757:i32)
                                n635 = local read "deviation y5"() -> (w749:dbl)
                                n636 = Divide(x=w757, y=w755) -> (x/y=w756:dbl)
                                n637 = Add(x=w756, y=w749) -> (x+y=w748:dbl)
                                n638 = local write "deviation y5"(w748) -> ()
                                }
                                }
                                frame #1 {
                                n639 = local read "deviation y3 min"() -> (w798:dbl)
                                n640 = local read "deviation y5 min"() -> (w795:dbl)
                                n641 = local read "deviation x5 min"() -> (w801:dbl)
                                n642 = local read "deviation x3 min"() -> (w804:dbl)
                                n643 = local read "deviation y5"() -> (w796:dbl)
                                n644 = local read "deviation y3"() -> (w799:dbl)
                                n645 = local read "deviation x5"() -> (w802:dbl)
                                n646 = local read "deviation x3"() -> (w805:dbl)
                                n647 = Max & Min(x=w799, y=w798) -> (min(x,y)=w797:dbl)  [unwired: 1 out]
                                n648 = Max & Min(x=w796, y=w795) -> (min(x,y)=w794:dbl)  [unwired: 1 out]
                                n649 = Max & Min(x=w805, y=w804) -> (min(x,y)=w803:dbl)  [unwired: 1 out]
                                n650 = Max & Min(x=w802, y=w801) -> (min(x,y)=w800:dbl)  [unwired: 1 out]
                                n651 = local write "deviation y3 min"(w797) -> ()
                                n652 = local write "deviation y5 min"(w794) -> ()
                                n653 = local write "deviation x3 min"(w803) -> ()
                                n654 = local write "deviation x5 min"(w800) -> ()
                                }
                                }
                                }
                              }
                              frame #5 {
                                n655 = local read "error x3"() -> (w808:bool)
                                n656 = local read "error y3"() -> (w809:bool)
                                n657 = local read "error x5"() -> (w807:bool)
                                n658 = local read "error y5"() -> (w806:bool)
                                n659 = case shown="True" w808 {
                                frame False {
                                n660 = local read "deviation precision err x 3"() -> (w829:dbl)
                                n661 = local read "deviation x3 min"() -> (w830:dbl)
                                n662 = Greater Or Equal?(x=w830, y=w829) -> (x >= y?=w828:bool)
                                n663 = local write "error x3"(w828) -> ()
                                n664 = local write "deviation error x3"(w828) -> ()
                                }
                                frame True {
                                n665 = local read "deviation precision err x 3"() -> (w833:dbl)
                                n666 = local read "deviation x3 min"() -> (w832:dbl)
                                n667 = Greater Or Equal?(x=w832, y=w833) -> (x >= y?=w831:bool)
                                n668 = local write "deviation error x3"(w831) -> ()
                                }
                                }
                                n669 = case shown="True" w809 {
                                frame False {
                                n670 = local read "deviation precision err y 3"() -> (w823:dbl)
                                n671 = local read "deviation y3 min"() -> (w824:dbl)
                                n672 = Greater Or Equal?(x=w824, y=w823) -> (x >= y?=w822:bool)
                                n673 = local write "error y3"(w822) -> ()
                                n674 = local write "deviation error y3"(w822) -> ()
                                }
                                frame True {
                                n675 = local read "deviation precision err y 3"() -> (w827:dbl)
                                n676 = local read "deviation y3 min"() -> (w826:dbl)
                                n677 = Greater Or Equal?(x=w826, y=w827) -> (x >= y?=w825:bool)
                                n678 = local write "deviation error y3"(w825) -> ()
                                }
                                }
                                n679 = case shown="True" w807 {
                                frame False {
                                n680 = local read "deviation precision err x 5"() -> (w817:dbl)
                                n681 = local read "deviation x5 min"() -> (w818:dbl)
                                n682 = Greater Or Equal?(x=w818, y=w817) -> (x >= y?=w816:bool)
                                n683 = local write "error x5"(w816) -> ()
                                n684 = local write "deviation error x5"(w816) -> ()
                                }
                                frame True {
                                n685 = local read "deviation precision err x 5"() -> (w821:dbl)
                                n686 = local read "deviation x5 min"() -> (w820:dbl)
                                n687 = Greater Or Equal?(x=w820, y=w821) -> (x >= y?=w819:bool)
                                n688 = local write "deviation error x5"(w819) -> ()
                                }
                                }
                                n689 = case shown="True" w806 {
                                frame False {
                                n690 = local read "deviation precision err y 5"() -> (w811:dbl)
                                n691 = local read "deviation y5 min"() -> (w812:dbl)
                                n692 = Greater Or Equal?(x=w812, y=w811) -> (x >= y?=w810:bool)
                                n693 = local write "error y5"(w810) -> ()
                                n694 = local write "deviation error y5"(w810) -> ()
                                }
                                frame True {
                                n695 = local read "deviation precision err y 5"() -> (w815:dbl)
                                n696 = local read "deviation y5 min"() -> (w814:dbl)
                                n697 = Greater Or Equal?(x=w814, y=w815) -> (x >= y?=w813:bool)
                                n698 = local write "deviation error y5"(w813) -> ()
                                }
                                }
                              }
                              frame #6 {
                                n699 = local read "deviation error y3"() -> (w837:bool)
                                n700 = local read "deviation error x3"() -> (w838:bool)
                                n701 = local read "max/min y3"() -> (w840:bool)
                                n702 = local read "max/min x3"() -> (w839:bool)
                                n703 = Or(x=w839, y=w840) -> (x .or. y?=w835:bool)
                                n704 = Or(x=w838, y=w837) -> (x .or. y?=w836:bool)
                                n705 = Or(x=w835, y=w836) -> (x .or. y?=w834:bool)
                                n706 = case shown="True" w834 {
                                frame False {
                                }
                                frame True {
                                n707 = local read "gathered err x 3"() -> (w888:i16[])
                                n708 = local read "gathered err y 3"() -> (w887:i16[])
                                n709 = local read "gathered err x 5"() -> (w852:i16[])
                                n710 = local read "gathered err y 5"() -> (w853:i16[])
                                n711 = local read "deviation x3 min"() -> (w882:dbl)
                                n712 = local read "deviation y3 min"() -> (w883:dbl)
                                n713 = local read "deviation x5 min"() -> (w855:dbl)
                                n714 = local read "deviation y5 min"() -> (w854:dbl)
                                n715 = local read "trigger count"() -> (w884:i16)
                                n716 = call "Convert to Dynamic Data3"("Array"=w888) -> ("Dynamic Data Type"=w896:dynamicdata)  [unwired: 3 in]
                                n717 = call "Convert to Dynamic Data4"("Array"=w887) -> ("Dynamic Data Type"=w895:dynamicdata)  [unwired: 3 in]
                                n718 = call "Convert to Dynamic Data7"("Array"=w852) -> ("Dynamic Data Type"=w850:dynamicdata)  [unwired: 3 in]
                                n719 = call "Convert to Dynamic Data8"("Array"=w853) -> ("Dynamic Data Type"=w851:dynamicdata)  [unwired: 3 in]
                                n720 = local read "max y5 now"() -> (w858:i16)
                                n721 = local read "max y3 now"() -> (w879:i16)
                                n722 = local read "max x3 now"() -> (w881:i16)
                                n723 = local read "max x5 now"() -> (w856:i16)
                                n724 = local read "min x3 now"() -> (w880:i16)
                                n725 = local read "min y3 now"() -> (w878:i16)
                                n726 = local read "min x5 now"() -> (w857:i16)
                                n727 = local read "min y5 now"() -> (w859:i16)
                                n728 = xnode "Set Dynamic Data Attributes"("Signals In"=w896, "Signal Name"="err x3    ") -> ("Signals Out"=w893:dynamicdata)  [unwired: 2 in, 1 out]
                                n729 = xnode "Set Dynamic Data Attributes"("Signals In"=w895, "Signal Name"="err y3    ") -> ("Signals Out"=w894:dynamicdata)  [unwired: 2 in, 1 out]
                                n730 = xnode "Set Dynamic Data Attributes"("Signals In"=w883, "Signal Name"="deviation y3") -> ("Signals Out"=w885:dynamicdata)  [unwired: 2 in, 1 out]
                                n731 = xnode "Set Dynamic Data Attributes"("Signals In"=w884, "Signal Name"="trigger count") -> ("Signals Out"=w868:dynamicdata)  [unwired: 2 in, 1 out]
                                n732 = xnode "Set Dynamic Data Attributes"("Signals In"=w850, "Signal Name"="err x5    ") -> ("Signals Out"=w849:dynamicdata)  [unwired: 2 in, 1 out]
                                n733 = xnode "Set Dynamic Data Attributes"("Signals In"=w851, "Signal Name"="err y5    ") -> ("Signals Out"=w848:dynamicdata)  [unwired: 2 in, 1 out]
                                n734 = xnode "Set Dynamic Data Attributes"("Signals In"=w881, "Signal Name"="max err x3") -> ("Signals Out"=w892:dynamicdata)  [unwired: 2 in, 1 out]
                                n735 = xnode "Set Dynamic Data Attributes"("Signals In"=w880, "Signal Name"="min err x3") -> ("Signals Out"=w891:dynamicdata)  [unwired: 2 in, 1 out]
                                n736 = xnode "Set Dynamic Data Attributes"("Signals In"=w879, "Signal Name"="max err y3") -> ("Signals Out"=w890:dynamicdata)  [unwired: 2 in, 1 out]
                                n737 = xnode "Set Dynamic Data Attributes"("Signals In"=w878, "Signal Name"="min err y3") -> ("Signals Out"=w889:dynamicdata)  [unwired: 2 in, 1 out]
                                n738 = xnode "Set Dynamic Data Attributes"("Signals In"=w882, "Signal Name"="deviation x3") -> ("Signals Out"=w886:dynamicdata)  [unwired: 2 in, 1 out]
                                n739 = xnode "Set Dynamic Data Attributes"("Signals In"=w856, "Signal Name"="max err x5") -> ("Signals Out"=w847:dynamicdata)  [unwired: 2 in, 1 out]
                                n740 = xnode "Set Dynamic Data Attributes"("Signals In"=w857, "Signal Name"="min err x5") -> ("Signals Out"=w846:dynamicdata)  [unwired: 2 in, 1 out]
                                n741 = xnode "Set Dynamic Data Attributes"("Signals In"=w858, "Signal Name"="max err y5") -> ("Signals Out"=w845:dynamicdata)  [unwired: 2 in, 1 out]
                                n742 = xnode "Set Dynamic Data Attributes"("Signals In"=w859, "Signal Name"="min err y5") -> ("Signals Out"=w844:dynamicdata)  [unwired: 2 in, 1 out]
                                n743 = xnode "Set Dynamic Data Attributes"("Signals In"=w855, "Signal Name"="deviation x5") -> ("Signals Out"=w843:dynamicdata)  [unwired: 2 in, 1 out]
                                n744 = xnode "Set Dynamic Data Attributes"("Signals In"=w854, "Signal Name"="deviation y5") -> ("Signals Out"=w842:dynamicdata)  [unwired: 2 in, 1 out]
                                n745 = Merge Signals(w893, w894, w892, w891, w890, w889, w886, w885, w868, w849, w848, w847, w846, w845, w844, w843, w842) -> (w897:dynamicdata)
                                n746 = call "Write To Measurement File2"("Signals"=w897, "Filename"="Filename errors") -> ()  [unwired: 15 in, 3 out]
                                }
                                }
                              }
                              frame #7 {
                                n747 = local read "gathered err x 3"() -> (w1146:i16[])
                                n748 = local read "gathered err y 3"() -> (w1147:i16[])
                                n749 = local read "gathered err x 5"() -> (w1182:i16[])
                                n750 = local read "gathered err y 5"() -> (w1181:i16[])
                                n751 = local read "deviation x3 min"() -> (w1152:dbl)
                                n752 = local read "deviation y3 min"() -> (w1151:dbl)
                                n753 = local read "deviation x5 min"() -> (w1179:dbl)
                                n754 = local read "deviation y5 min"() -> (w1180:dbl)
                                n755 = local read "trigger count"() -> (w1150:i16)
                                n756 = call "Convert to Dynamic Data5"("Array"=w1146) -> ("Dynamic Data Type"=w1138:dynamicdata)  [unwired: 3 in]
                                n757 = call "Convert to Dynamic Data6"("Array"=w1147) -> ("Dynamic Data Type"=w1139:dynamicdata)  [unwired: 3 in]
                                n758 = call "Convert to Dynamic Data9"("Array"=w1182) -> ("Dynamic Data Type"=w1184:dynamicdata)  [unwired: 3 in]
                                n759 = call "Convert to Dynamic Data10"("Array"=w1181) -> ("Dynamic Data Type"=w1183:dynamicdata)  [unwired: 3 in]
                                n760 = local read "max y5 now"() -> (w1176:i16)
                                n761 = local read "max y3 now"() -> (w1155:i16)
                                n762 = local read "max x3 now"() -> (w1153:i16)
                                n763 = local read "max x5 now"() -> (w1178:i16)
                                n764 = local read "min x3 now"() -> (w1154:i16)
                                n765 = local read "min y3 now"() -> (w1156:i16)
                                n766 = local read "min x5 now"() -> (w1177:i16)
                                n767 = local read "min y5 now"() -> (w1175:i16)
                                n768 = xnode "Set Dynamic Data Attributes"("Signals In"=w1138, "Signal Name"="err x3    ") -> ("Signals Out"=w1141:dynamicdata)  [unwired: 2 in, 1 out]
                                n769 = xnode "Set Dynamic Data Attributes"("Signals In"=w1139, "Signal Name"="err y3    ") -> ("Signals Out"=w1140:dynamicdata)  [unwired: 2 in, 1 out]
                                n770 = xnode "Set Dynamic Data Attributes"("Signals In"=w1151, "Signal Name"="deviation y3") -> ("Signals Out"=w1149:dynamicdata)  [unwired: 2 in, 1 out]
                                n771 = xnode "Set Dynamic Data Attributes"("Signals In"=w1150, "Signal Name"="trigger count") -> ("Signals Out"=w1166:dynamicdata)  [unwired: 2 in, 1 out]
                                n772 = xnode "Set Dynamic Data Attributes"("Signals In"=w1184, "Signal Name"="err x5    ") -> ("Signals Out"=w1185:dynamicdata)  [unwired: 2 in, 1 out]
                                n773 = xnode "Set Dynamic Data Attributes"("Signals In"=w1183, "Signal Name"="err y5    ") -> ("Signals Out"=w1186:dynamicdata)  [unwired: 2 in, 1 out]
                                n774 = xnode "Set Dynamic Data Attributes"("Signals In"=w1153, "Signal Name"="max err x3") -> ("Signals Out"=w1142:dynamicdata)  [unwired: 2 in, 1 out]
                                n775 = xnode "Set Dynamic Data Attributes"("Signals In"=w1154, "Signal Name"="min err x3") -> ("Signals Out"=w1143:dynamicdata)  [unwired: 2 in, 1 out]
                                n776 = xnode "Set Dynamic Data Attributes"("Signals In"=w1155, "Signal Name"="max err y3") -> ("Signals Out"=w1144:dynamicdata)  [unwired: 2 in, 1 out]
                                n777 = xnode "Set Dynamic Data Attributes"("Signals In"=w1156, "Signal Name"="min err y3") -> ("Signals Out"=w1145:dynamicdata)  [unwired: 2 in, 1 out]
                                n778 = xnode "Set Dynamic Data Attributes"("Signals In"=w1152, "Signal Name"="deviation x3") -> ("Signals Out"=w1148:dynamicdata)  [unwired: 2 in, 1 out]
                                n779 = xnode "Set Dynamic Data Attributes"("Signals In"=w1178, "Signal Name"="max err x5") -> ("Signals Out"=w1187:dynamicdata)  [unwired: 2 in, 1 out]
                                n780 = xnode "Set Dynamic Data Attributes"("Signals In"=w1177, "Signal Name"="min err x5") -> ("Signals Out"=w1188:dynamicdata)  [unwired: 2 in, 1 out]
                                n781 = xnode "Set Dynamic Data Attributes"("Signals In"=w1176, "Signal Name"="max err y5") -> ("Signals Out"=w1189:dynamicdata)  [unwired: 2 in, 1 out]
                                n782 = xnode "Set Dynamic Data Attributes"("Signals In"=w1175, "Signal Name"="min err y5") -> ("Signals Out"=w1190:dynamicdata)  [unwired: 2 in, 1 out]
                                n783 = xnode "Set Dynamic Data Attributes"("Signals In"=w1179, "Signal Name"="deviation x5") -> ("Signals Out"=w1191:dynamicdata)  [unwired: 2 in, 1 out]
                                n784 = xnode "Set Dynamic Data Attributes"("Signals In"=w1180, "Signal Name"="deviation y5") -> ("Signals Out"=w1192:dynamicdata)  [unwired: 2 in, 1 out]
                                n785 = Merge Signals(w1141, w1140, w1142, w1143, w1144, w1145, w1148, w1149, w1166, w1185, w1186, w1187, w1188, w1189, w1190, w1191, w1192) -> (w1137:dynamicdata)
                                n786 = call "Write To Measurement File3"("Signals"=w1137, "Filename"="Filename history") -> ()  [unwired: 15 in, 3 out]
                              }
                            }
                          }
                        }
                      }
                      frame #4 {
                        n787 = local read "number of elements"() -> (w1435:u32)
                        n788 = local read "end trigger index"() -> (w1433:i32)
                        n789 = local read "error x 5 now"() -> (w1437:i16[])
                        n790 = local read "error y 5 now"() -> (w1432:i16[])
                        n791 = Subtract(x=w1435, y=w1433) -> (x-y=w1434:u32)
                        n792 = Array Subset(array=w1437, index=w1433, length=w1434) -> (w1436:i16[])
                        n793 = Array Subset(array=w1432, index=w1433, length=w1434) -> (w1431:i16[])
                        n794 = for {
                          N: w1434 -> [_]
                          tunnel: w1436 -> [w1447]
                          tunnel: w1431 -> [w1446]
                          i -> [w1438]
                          stop <- w1448 stop-if-true
                          n795 = Index Array(array=w1447, index=w1438) -> (element=w1441:i16)
                          n796 = Index Array(array=w1446, index=w1438) -> (element=w1440:i16)
                          n797 = local read "x5 0 level"() -> (w1443:i16)
                          n798 = local read "y5 0 level"() -> (w1444:i16)
                          n799 = local read "trigger treshold"() -> (w1445:i16)
                          n800 = Subtract(x=w1441, y=w1443) -> (x-y=w1442:i16)
                          n801 = Subtract(x=w1440, y=w1444) -> (x-y=w1439:i16)
                          n802 = local write "trigger index"(w1438) -> ()
                          n803 = Greater?(x=w1442, y=w1445) -> (0:w1455:bool)
                          n804 = Negate(x=w1445) -> (-x=w1456:i16)
                          n805 = Negate(x=w1445) -> (-x=w1453:i16)
                          n806 = Greater?(x=w1439, y=w1445) -> (0:w1452:bool)
                          n807 = Less?(x=w1442, y=w1456) -> (x < y?=w1454:bool)
                          n808 = Less?(x=w1439, y=w1453) -> (x < y?=w1451:bool)
                          n809 = Or(x=w1455, y=w1454) -> (x .or. y?=w1449:bool)
                          n810 = Or(x=w1452, y=w1451) -> (x .or. y?=w1450:bool)
                          n811 = Or(x=w1449, y=w1450) -> (x .or. y?=w1448:bool)
                          n812 = local write "trigger"(w1448) -> ()
                        }
                      }
                      frame #5 {
                        n813 = local read "trigger"() -> (w1457:bool)
                        n814 = case shown="True" w1457 {
                          frame False {
                          }
                          frame True {
                            n815 = flat-sequence {
                              frame #0 {
                                n816 = local read "reset"() -> (w1458:i16[])
                                n817 = local read "trigger count"() -> (w1460:i16)
                                n818 = local write "gathered err x 3"(w1458) -> ()
                                n819 = local write "gathered err y 3"(w1458) -> ()
                                n820 = local write "gathered err x 5"(w1458) -> ()
                                n821 = local write "gathered err y 5"(w1458) -> ()
                                n822 = Increment(x=w1460) -> (x+1=w1459:i16)
                                n823 = local write "trigger count"(w1459) -> ()
                              }
                              frame #1 {
                                n824 = local read "number of pts after trigger stops"() -> (w1468:i32)
                                n825 = local read "number of elements"() -> (w1463:u32)
                                n826 = Divide(x=w1468, y=w1463) -> (x/y=w1470:dbl)
                                n827 = Round Toward -Infinity(1:w1470) -> (0:w1461:dbl)
                                n828 = Multiply(x=w1461, y=w1463) -> (x*y=w1469:dbl)
                                n829 = local write "cycles to complete"(w1461) -> ()
                                n830 = local read "trigger index"() -> (w1466:i32)
                                n831 = Subtract(x=w1468, y=w1469) -> (x-y=w1467:dbl)
                                n832 = Add(x=w1467, y=w1466) -> (x+y=w1464:dbl)
                                n833 = Greater Or Equal?(x=w1464, y=w1463) -> (x >= y?=w1465:bool)
                                n834 = case shown="False" w1465 {
                                tunnel: w1464 -> [w1471 w1474]
                                tunnel: w1463 -> [_ w1473]
                                tunnel: [w1471 w1472] -> w1462
                                frame False {
                                }
                                frame True {
                                n835 = Subtract(x=w1474, y=w1473) -> (x-y=w1472:dbl)
                                n836 = local read "cycles to complete"() -> (w1476:i32)
                                n837 = Increment(x=w1476) -> (x+1=w1475:i32)
                                n838 = local write "cycles to complete"(w1475) -> ()
                                }
                                }
                                n839 = local write "end trigger index"(w1462) -> ()
                              }
                              frame #2 {
                                n840 = local read "cycles to complete"() -> (w1489:i32)
                                n841 = local read "number of elements"() -> (w1491:u32)
                                n842 = local read "number of elements"() -> (w1486:u32)
                                n843 = local read "trigger index"() -> (w1490:i32)
                                n844 = local read "trigger index"() -> (w1487:i32)
                                n845 = local read "error y 3 now"() -> (w1493:i16[])
                                n846 = local read "error y 5 now"() -> (w1484:i16[])
                                n847 = local read "error x 3 now"() -> (w1492:i16[])
                                n848 = local read "error x 5 now"() -> (w1485:i16[])
                                n849 = Decrement(x=w1489) -> (x-1=w1488:i32)
                                n850 = local read "gathered err y 3"() -> (w1495:i16[])
                                n851 = local read "gathered err x 3"() -> (w1494:i16[])
                                n852 = local read "gathered err y 5"() -> (w1482:i16[])
                                n853 = local read "gathered err x 5"() -> (w1483:i16[])
                                n854 = Subtract(x=w1491, y=w1490) -> (x-y=w1500:u32)
                                n855 = Subtract(x=w1486, y=w1487) -> (x-y=w1477:u32)
                                n856 = local write "cycles to complete"(w1488) -> ()
                                n857 = Array Subset(array=w1493, index=w1490, length=w1500) -> (w1498:i16[])
                                n858 = Array Subset(array=w1492, index=w1490, length=w1500) -> (w1499:i16[])
                                n859 = Array Subset(array=w1484, index=w1487, length=w1477) -> (w1479:i16[])
                                n860 = Array Subset(array=w1485, index=w1487, length=w1477) -> (w1478:i16[])
                                n861 = Build Array (concatenate)(w1495, w1498) -> (w1497:i16[])
                                n862 = Build Array (concatenate)(w1494, w1499) -> (w1496:i16[])
                                n863 = Build Array (concatenate)(w1482, w1479) -> (w1480:i16[])
                                n864 = Build Array (concatenate)(w1483, w1478) -> (w1481:i16[])
                                n865 = local write "gathered err y 3"(w1497) -> ()
                                n866 = local write "gathered err x 3"(w1496) -> ()
                                n867 = local write "gathered err y 5"(w1480) -> ()
                                n868 = local write "gathered err x 5"(w1481) -> ()
                              }
                            }
                          }
                        }
                      }
                    }
                  }
                }
              }
            }
          }
        }
      }
    }
  }
  n869 = xnode "Close FPGA VI Reference"("FPGA VI Reference In"=w16, "error in"=w15) -> ()  [unwired: 1 out]
